vi "运维调试_质控单元.vi"() -> ()   [LabVIEW 2016, in "质控单元.lvlib"]
uses:
  <vilib>/Utility/miscctls.llb/LVPointTypeDef.ctl
  <vilib>/Analysis/6fits.llb/Curve Fitting Criteria.ctl
  <vilib>/Plasmionique/MB Master/MB_Master_Serial/MB_Master_Serial.lvclass
  C:/Program Files (x86)/National Instruments/LabVIEW 2016/vi.lib/Plasmionique/MB Master/MB_Master/MB_Master.lvclass
  <vilib>/Utility/config.llb/Write Key (I32).vi
  <vilib>/Utility/config.llb/Write Key (Double).vi
  <vilib>/Utility/config.llb/Write Key (Boolean).vi
  <vilib>/Utility/config.llb/Write Key (U32).vi
  <vilib>/Utility/config.llb/Read Key (I32).vi
  <vilib>/Utility/config.llb/Read Key (Double).vi
  <vilib>/Utility/config.llb/Read Key (Boolean).vi
  <vilib>/Utility/config.llb/Read Key (U32).vi
  <vilib>/Plasmionique/MB Master/MB Master.lvlib
  <vilib>/ptbypt/NI_PtbyPt.lvlib
  <vilib>/Utility/config.llb/NI_LVConfig.lvlib
  <vilib>/Analysis/NI_AALPro.lvlib
panel:
  out "CODMn质控中断报警":bool
  out "总磷质控中断报警":bool
  out "总氮质控中断报警":bool
  out "氨氮质控中断报警":bool
  in  "报警清除":bool
  in  "CODMn量程选择":enum32{"H", "L", "AUTO"}(ring)
  in  "CODMn加标回收启动":bool
  in  "总磷总氮加标回收启动":bool
  in  "氨氮加标回收启动":bool
  in  "总磷量程选择":enum32{"H", "L", "AUTO"}(ring)=enum."AUTO"
  in  "总氮量程选择":enum32{"H", "L", "AUTO"}(ring)=enum."AUTO"
  in  "氨氮量程选择":enum32{"H", "L", "AUTO"}(ring)=enum."AUTO"
  out "COD超时报警":bool
  out "总磷总氮超时报警":bool
  out "氨氮进样超时报警":bool
  out "簇":T1
  out "通讯指示灯3":bool
  out "通讯指示灯2":bool
  out "通讯指示灯1":bool
  in  "模块选择 3":bool
  in  "模块选择 2":bool
  in  "模块选择":bool
  in  "枚举":enum16{"柱塞泵1", "柱塞泵2", "柱塞泵3"}(ring)
  in  "启用":bool
  in  "B 3":dbl caption="B3"
  in  "K 3":dbl caption="K3"
  in  "B 2":dbl caption="B2"
  in  "K 2":dbl caption="K2"
  in  "B":dbl caption="B1"
  in  "K":dbl caption="K1"
  out "r^2":dbl format="%_6g"
  out "拟合方程":string
  in  "实际体积 5":dbl
  in  "标准体积 5":dbl
  in  "实际体积 4":dbl
  in  "标准体积 4":dbl
  in  "实际体积 3":dbl
  in  "实际体积 2":dbl
  in  "实际体积 1":dbl
  in  "标准体积 3":dbl
  in  "标准体积 2":dbl
  in  "标准体积 1":dbl
  in  "读取":bool
  in  "柱塞泵3":bool
  in  "柱塞泵2":bool
  in  "柱塞泵1":bool
  in  "注出体积选择":u16(ring) items=["0.1mL", "0.3mL", "0.5mL", "0.8mL", "1.0mL"]
  out "Serial Config":T2={"baud rate (bps)"=115200, "stop bits"=10, "parity"=0, "flow control"=0, "timeout"=100, "retries"=1} {"stop bits" items=["1.0"=10, "1.5"=15, "2.0"=20]; "parity" items=["None", "Odd", "Even", "Mark", "Space"]; "flow control" items=["None", "XON/XOFF", "RTS/CTS", "XON/XOFF & RTS/CTS", "DTR/DSR", "XON/XOFF & DTR/DSR"]}
  out "VISA Resource":refnum<visa-resource-name>="COM8"
  in  "背隙补偿步数 3":i32 min=0 max=2000
  in  "背隙补偿步数 2":i32 min=0 max=2000
  in  "写入":bool
  in  "背隙补偿步数":i32 min=0 max=2000
  out "总氮加标回收测完标志":bool
  out "启动模块":T3
  out "COD传感器故障报警":bool
  in  "总氮停止":bool
  in  "总氮排液":bool
  in  "总氮调试":bool
  out "总氮加标回收率":dbl caption="加标回收率" format="%.2f"
  out "总氮加标体积":dbl caption="加标体积" format="%.3f"
  out "总氮母液浓度":dbl caption="加标母液浓度" format="%.3f"
  out "总氮加标水杯定容体积":dbl caption="加标水杯定容体积" format="%.2f"
  out "总氮加标后水样浓度":dbl caption="加标后水样浓度" format="%.3f"
  out "总氮加标前水样浓度":dbl caption="加标前水样浓度" format="%.3f"
  out "总氮检出限":dbl caption="检出限" format="%.3f"
  out "总氮量程":dbl caption="量程" format="%.2f"
  out "总氮状态":u16(ring) caption="状态" items=["待机", "润洗", "进样", "等待取液", "排液"]
  in  "返回":bool
  in  "查看":bool
  out "直接启动":bool
  out "常规启动":bool
  out "总磷总氮传感器故障报警":bool
  out "氨氮传感器故障报警":bool
  out "columns":string[](array[string])
  out "data":T4
  out "氨氮加标回收测完标志":bool
  out "COD加标回收测完标志":bool
  out "总磷加标回收测完标志":bool
  out "COD平行样测完标志":bool
  out "氨氮总磷平行样测完标志":bool
  out "输出簇 2":T5
  out "常规启动 2":bool
  out "直接启动 2":bool
  out "启动模块 2":cluster{"氨氮1":bool, "总磷1":bool, " COD1":bool}
  in  "停止测量":bool
  out "输出簇":T6
  in  "加标回收":bool
  in  "平行样测试":bool
  in  "CODMn停止":bool
  in  "CODMn排液":bool
  in  "CODMn调试":bool
  in  "总磷停止":bool
  in  "总磷排液":bool
  in  "总磷调试":bool
  out "COD加标回收率":dbl caption="加标回收率" format="%.2f"
  out "COD加标体积":dbl caption="加标体积" format="%.3f"
  out "COD母液浓度":dbl caption="加标母液浓度" format="%.2f"
  out "COD加标水杯定容体积":dbl caption="加标水杯定容体积" format="%.2f"
  out "COD加标后水样浓度":dbl caption="加标后水样浓度" format="%.2f"
  out "COD加标前水样浓度":dbl caption="加标前水样浓度" format="%.2f"
  out "COD检出限":dbl caption="检出限" format="%.2f"
  out "COD量程":dbl caption="量程" format="%.2f"
  out "COD状态":u16(ring) caption="状态" items=["待机", "润洗", "进样", "等待取液", "排液"]
  out "总磷加标回收率":dbl caption="加标回收率" format="%.2f"
  out "总磷加标体积":dbl caption="加标体积" format="%.3f"
  out "总磷母液浓度":dbl caption="加标母液浓度" format="%.3f"
  out "总磷加标水杯定容体积":dbl caption="加标水杯定容体积" format="%.2f"
  out "总磷加标后水样浓度":dbl caption="加标后水样浓度" format="%.3f"
  out "总磷加标前水样浓度":dbl caption="加标前水样浓度" format="%.3f"
  out "总磷检出限":dbl caption="检出限" format="%.3f"
  out "总磷量程":dbl caption="量程" format="%.2f"
  out "总磷状态":u16(ring) caption="状态" items=["待机", "润洗", "进样", "等待取液", "排液"]
  out "氨氮加标回收率":dbl caption="加标回收率" format="%.2f"
  out "氨氮加标体积":dbl caption="加标体积" format="%.3f"
  out "氨氮母液浓度":dbl caption="加标母液浓度" format="%.3f"
  out "氨氮加标水杯定容体积":dbl caption="加标水杯定容体积" format="%.2f"
  out "氨氮加标后水样浓度":dbl caption="加标后水样浓度" format="%.3f"
  out "氨氮加标前水样浓度":dbl caption="加标前水样浓度" format="%.3f"
  out "氨氮检出限":dbl caption="检出限" format="%.3f"
  out "氨氮量程":dbl caption="量程" format="%.2f"
  out "氨氮状态":u16(ring) caption="状态" items=["待机", "润洗", "进样", "等待取液", "排液"]
  in  "氨氮停止":bool
  in  "氨氮排液":bool
  in  "氨氮调试":bool
  # "参数配置区"
  # "2000步等于1mL\n100步等于0.05mL\n20步等于0.01mL\n2步等于0.001mL\n（初始默认100步）"
  # "辅助计算区"
  # "状态显示区"
  # "总氮质控参数"
  # "%"
  # "mL"
  # "mg/L"
  # "mL"
  # "mg/L"
  # "mg/L"
  # "mg/L"
  # "mg/L"
  # "CODMn质控参数"
  # "%"
  # "mL"
  # "mg/L"
  # "mL"
  # "mg/L"
  # "mg/L"
  # "mg/L"
  # "mg/L"
  # "总磷质控参数"
  # "%"
  # "mL"
  # "mg/L"
  # "mL"
  # "mg/L"
  # "mg/L"
  # "mg/L"
  # "mg/L"
  # "氨氮质控参数"
  # "%"
  # "mL"
  # "mg/L"
  # "mL"
  # "mg/L"
  # "mg/L"
  # "mg/L"
  # "mg/L"
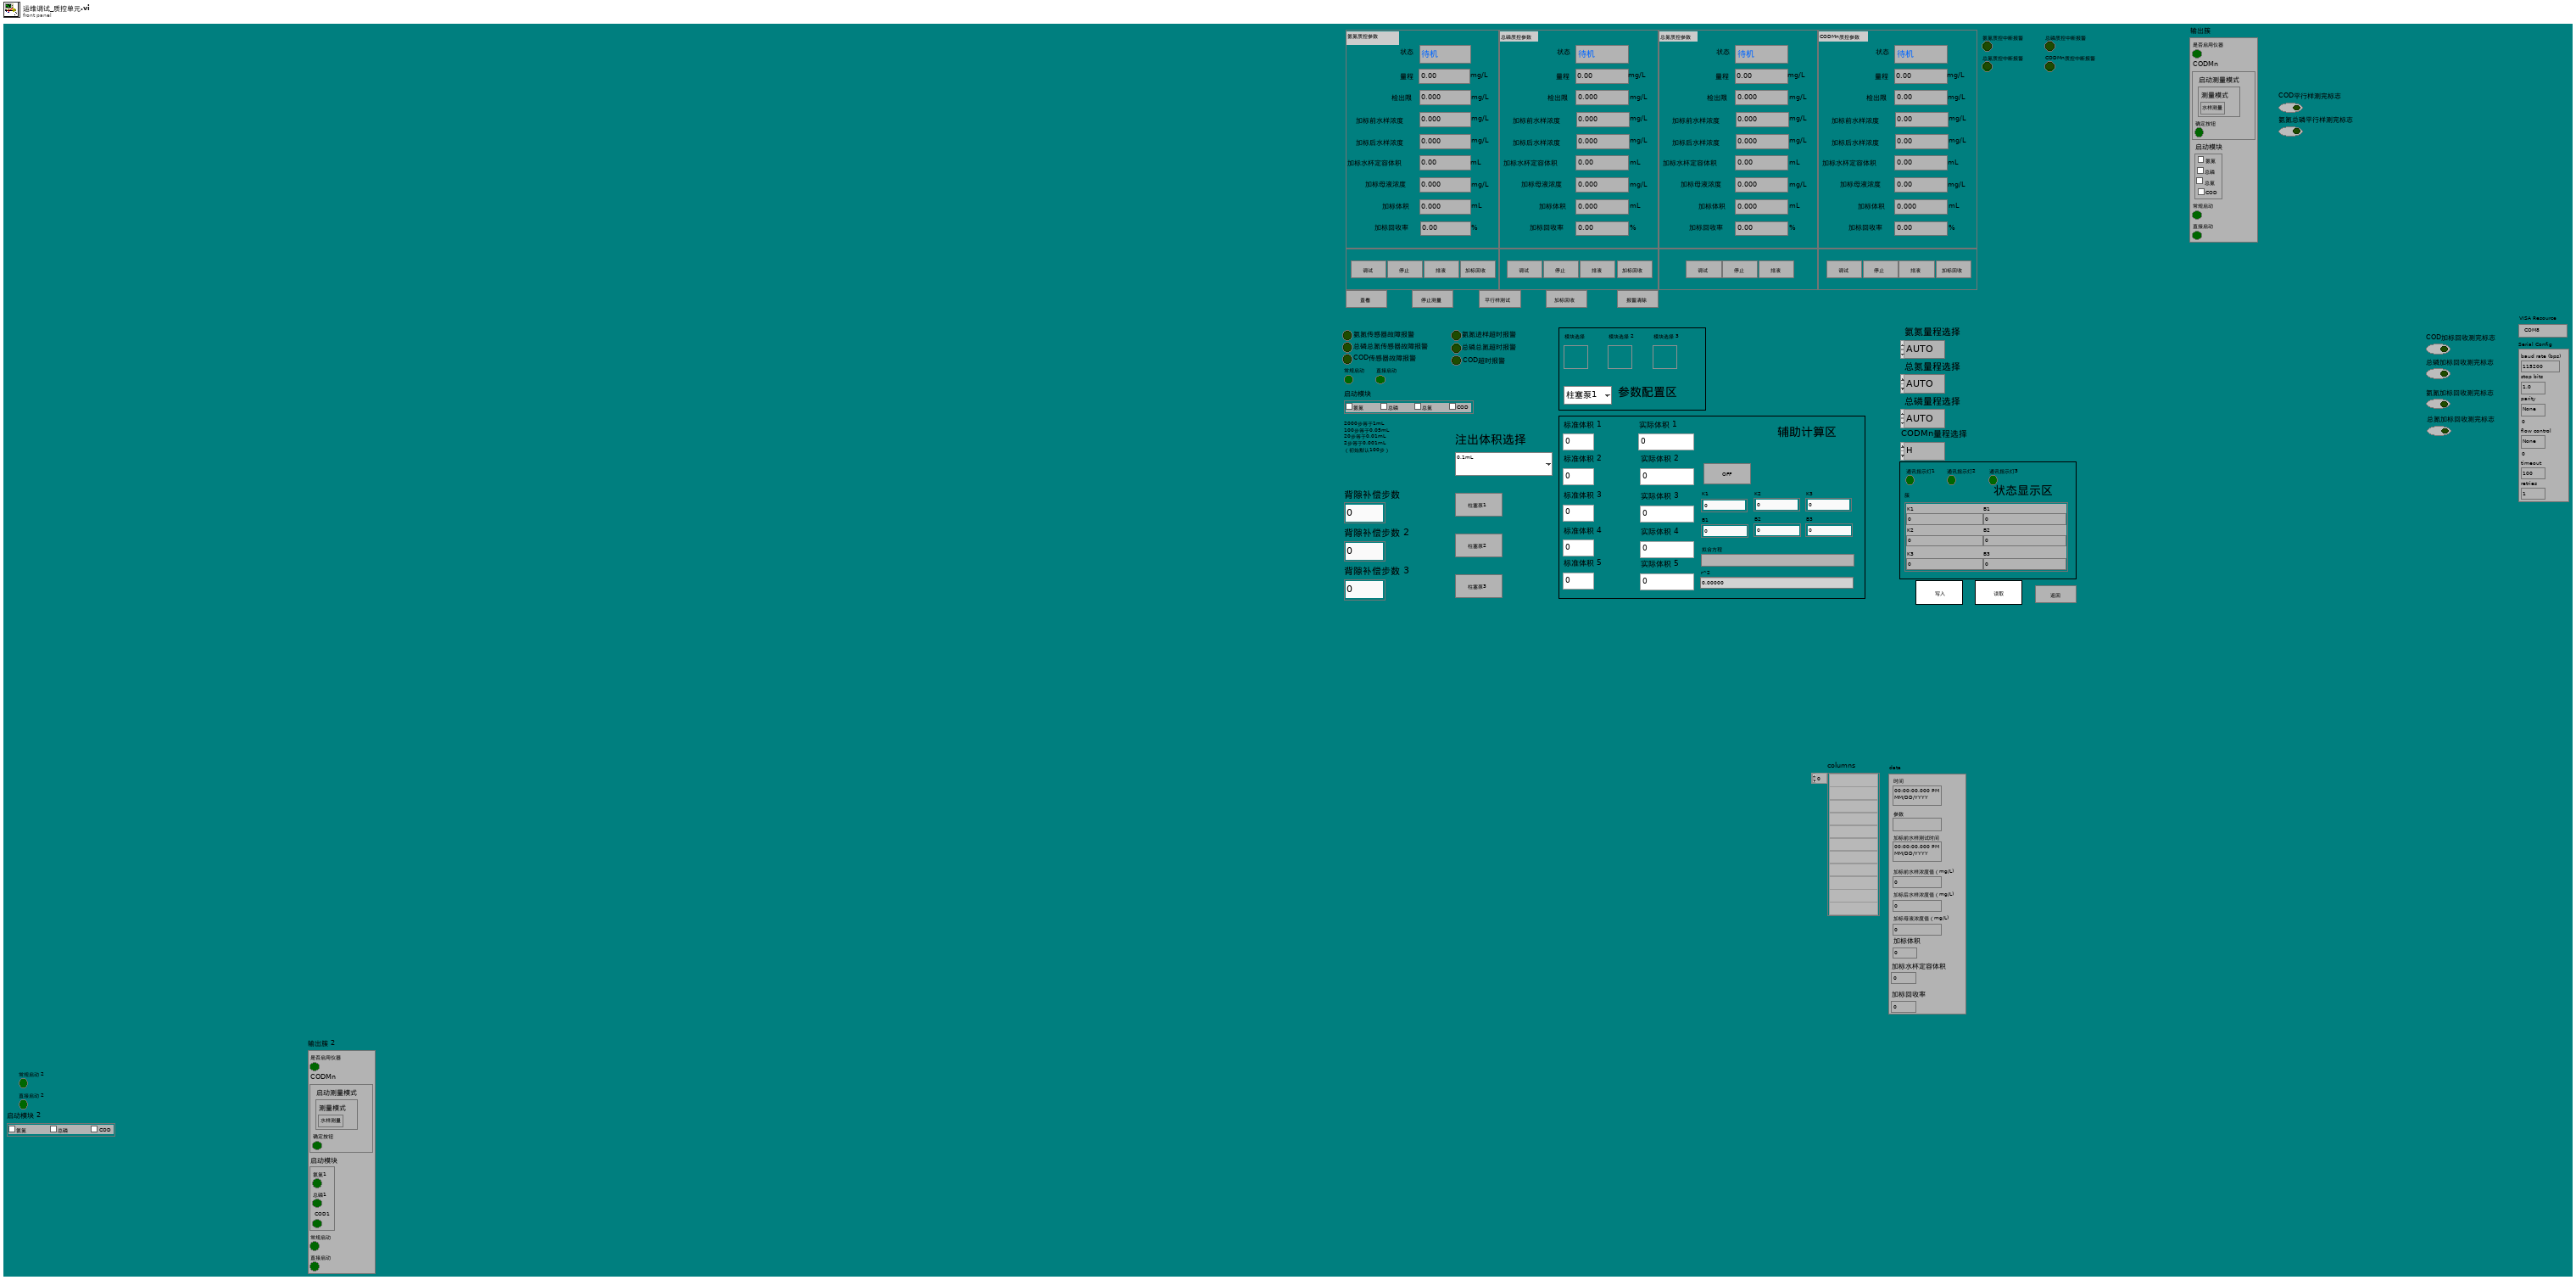
[diagram p1: front panel]
types:
  T1 = cluster{"K1":sgl, "B1":sgl, "K2":sgl, "B2":sgl, "K3":sgl, "B3":sgl}
  T2 = cluster{"baud rate (bps)":u32, "stop bits":u16, "parity":u16, "flow control":u16, "timeout":u32, "retries":i32}
  T3 = cluster{"氨氮":bool, "总磷":bool, "总氮":bool, "COD":bool}
  T4 = cluster{"时间":timestamp, "参数":string, "加标前水样测试时间":timestamp, "加标前水样浓度值（mg/L)":sgl, "加标后水样浓度值（mg/L)":sgl, "加标母液浓度值（mg/L)":sgl, "加标体积":dbl, "加标水杯定容体积":dbl, "加标回收率":dbl}
  T5 = cluster{"是否启用仪器":bool, "CODMn":cluster{"启动测量模式":cluster{"测量模式":enum16{"水样测量", "标样核查", "加标回收", "平行样", "校零", "校标"}}, "确定按钮":bool}, "启动模块":cluster{"氨氮1":bool, "总磷1":bool, " COD1":bool}, "常规启动":bool, "直接启动":bool}
  T6 = cluster{"是否启用仪器":bool, "CODMn":cluster{"启动测量模式":cluster{"测量模式":enum16{"水样测量", "标样核查", "加标回收", "平行样", "校零", "校标"}}, "确定按钮":bool}, "启动模块 3":cluster{"氨氮":bool, "总磷":bool, "总氮":bool, "COD":bool}, "常规启动":bool, "直接启动":bool}
  T7 = typedef "LVPointTypeDef.ctl" = cluster{"Horizontal":i16, "Vertical":i16}
  T8 = cluster{"量程":dbl, "检出限":dbl, "加标前水样浓度":dbl, "加标后水样浓度":dbl, "加标水杯定容体积":dbl, "加标母液浓度":dbl, "加标体积":dbl, "加标回收率":dbl}
  T9 = cluster{"因子编码":u32, "单位":u16, "标样参考值":sgl, "水样数据时间":timestamp, "水样实测值":sgl, "水样数据标识":string, "标样数据时间":timestamp, "标样实测值":sgl, "标样数据标识":string, "空白数据时间":timestamp, "空白实测值":sgl, "空白数据标识":string, "零点核查数据时间":timestamp, "零点核查实测值":sgl, "零点核查数据标识":string, "跨度核查数据时间":timestamp, "跨度核查实测值":sgl, "跨度核查数据标识":string, "加标回收数据时间":timestamp, "加标回收实测值":sgl, "加标回收数据标识":string, "平行样数据时间":timestamp, "平行样实测值":sgl, "平行样数据标识":string}
  T10 = cluster{"因子编码":u32, "单位":u16, "标样参考值":sgl, "水样数据时间":timestamp, "水样实测值":sgl, "水样数据标识":string, "标样数据时间":timestamp, "标样实测值":sgl, "标样数据标识":string, "空白数据时间":timestamp, "空白实测值":sgl, "空白数据标识":string, "零点核查数据时间":timestamp, "零点核查实测值":sgl, "零点核查数据标识":string, "跨度核查数据时间":timestamp, "跨度核查实测值":sgl, "跨度核查数据标识":string, "加标回收数据时间":timestamp, "加标回收实测值":sgl, "加标回收数据标识":string, "平行样数据时间":timestamp, "平行样实测值":sgl, "平行样数据标识":string, "F0":sgl, "F1":sgl, "F2":sgl, "F3":sgl, "F4":sgl, "F5":sgl, "F6":sgl, "F7":sgl, "温度":sgl, "湿度":sgl, "X值":sgl}
  T11 = enum8{"Enabled", "Disabled", "Disabled and Grayed Out"}
  T12 = typedef "NI_AALPro.lvlib/Curve Fitting Criteria.ctl" = u16
  T13 = typedef "NI_LVConfig.lvlib/Config Data RefNum.ctl" = refnum<k1>
  T14 = cluster{"命令":string, cluster{"starting address":u16, "holding register value":u16}}
  T15 = enum32{"Bad", "Idle", "Run top level", "Running"}
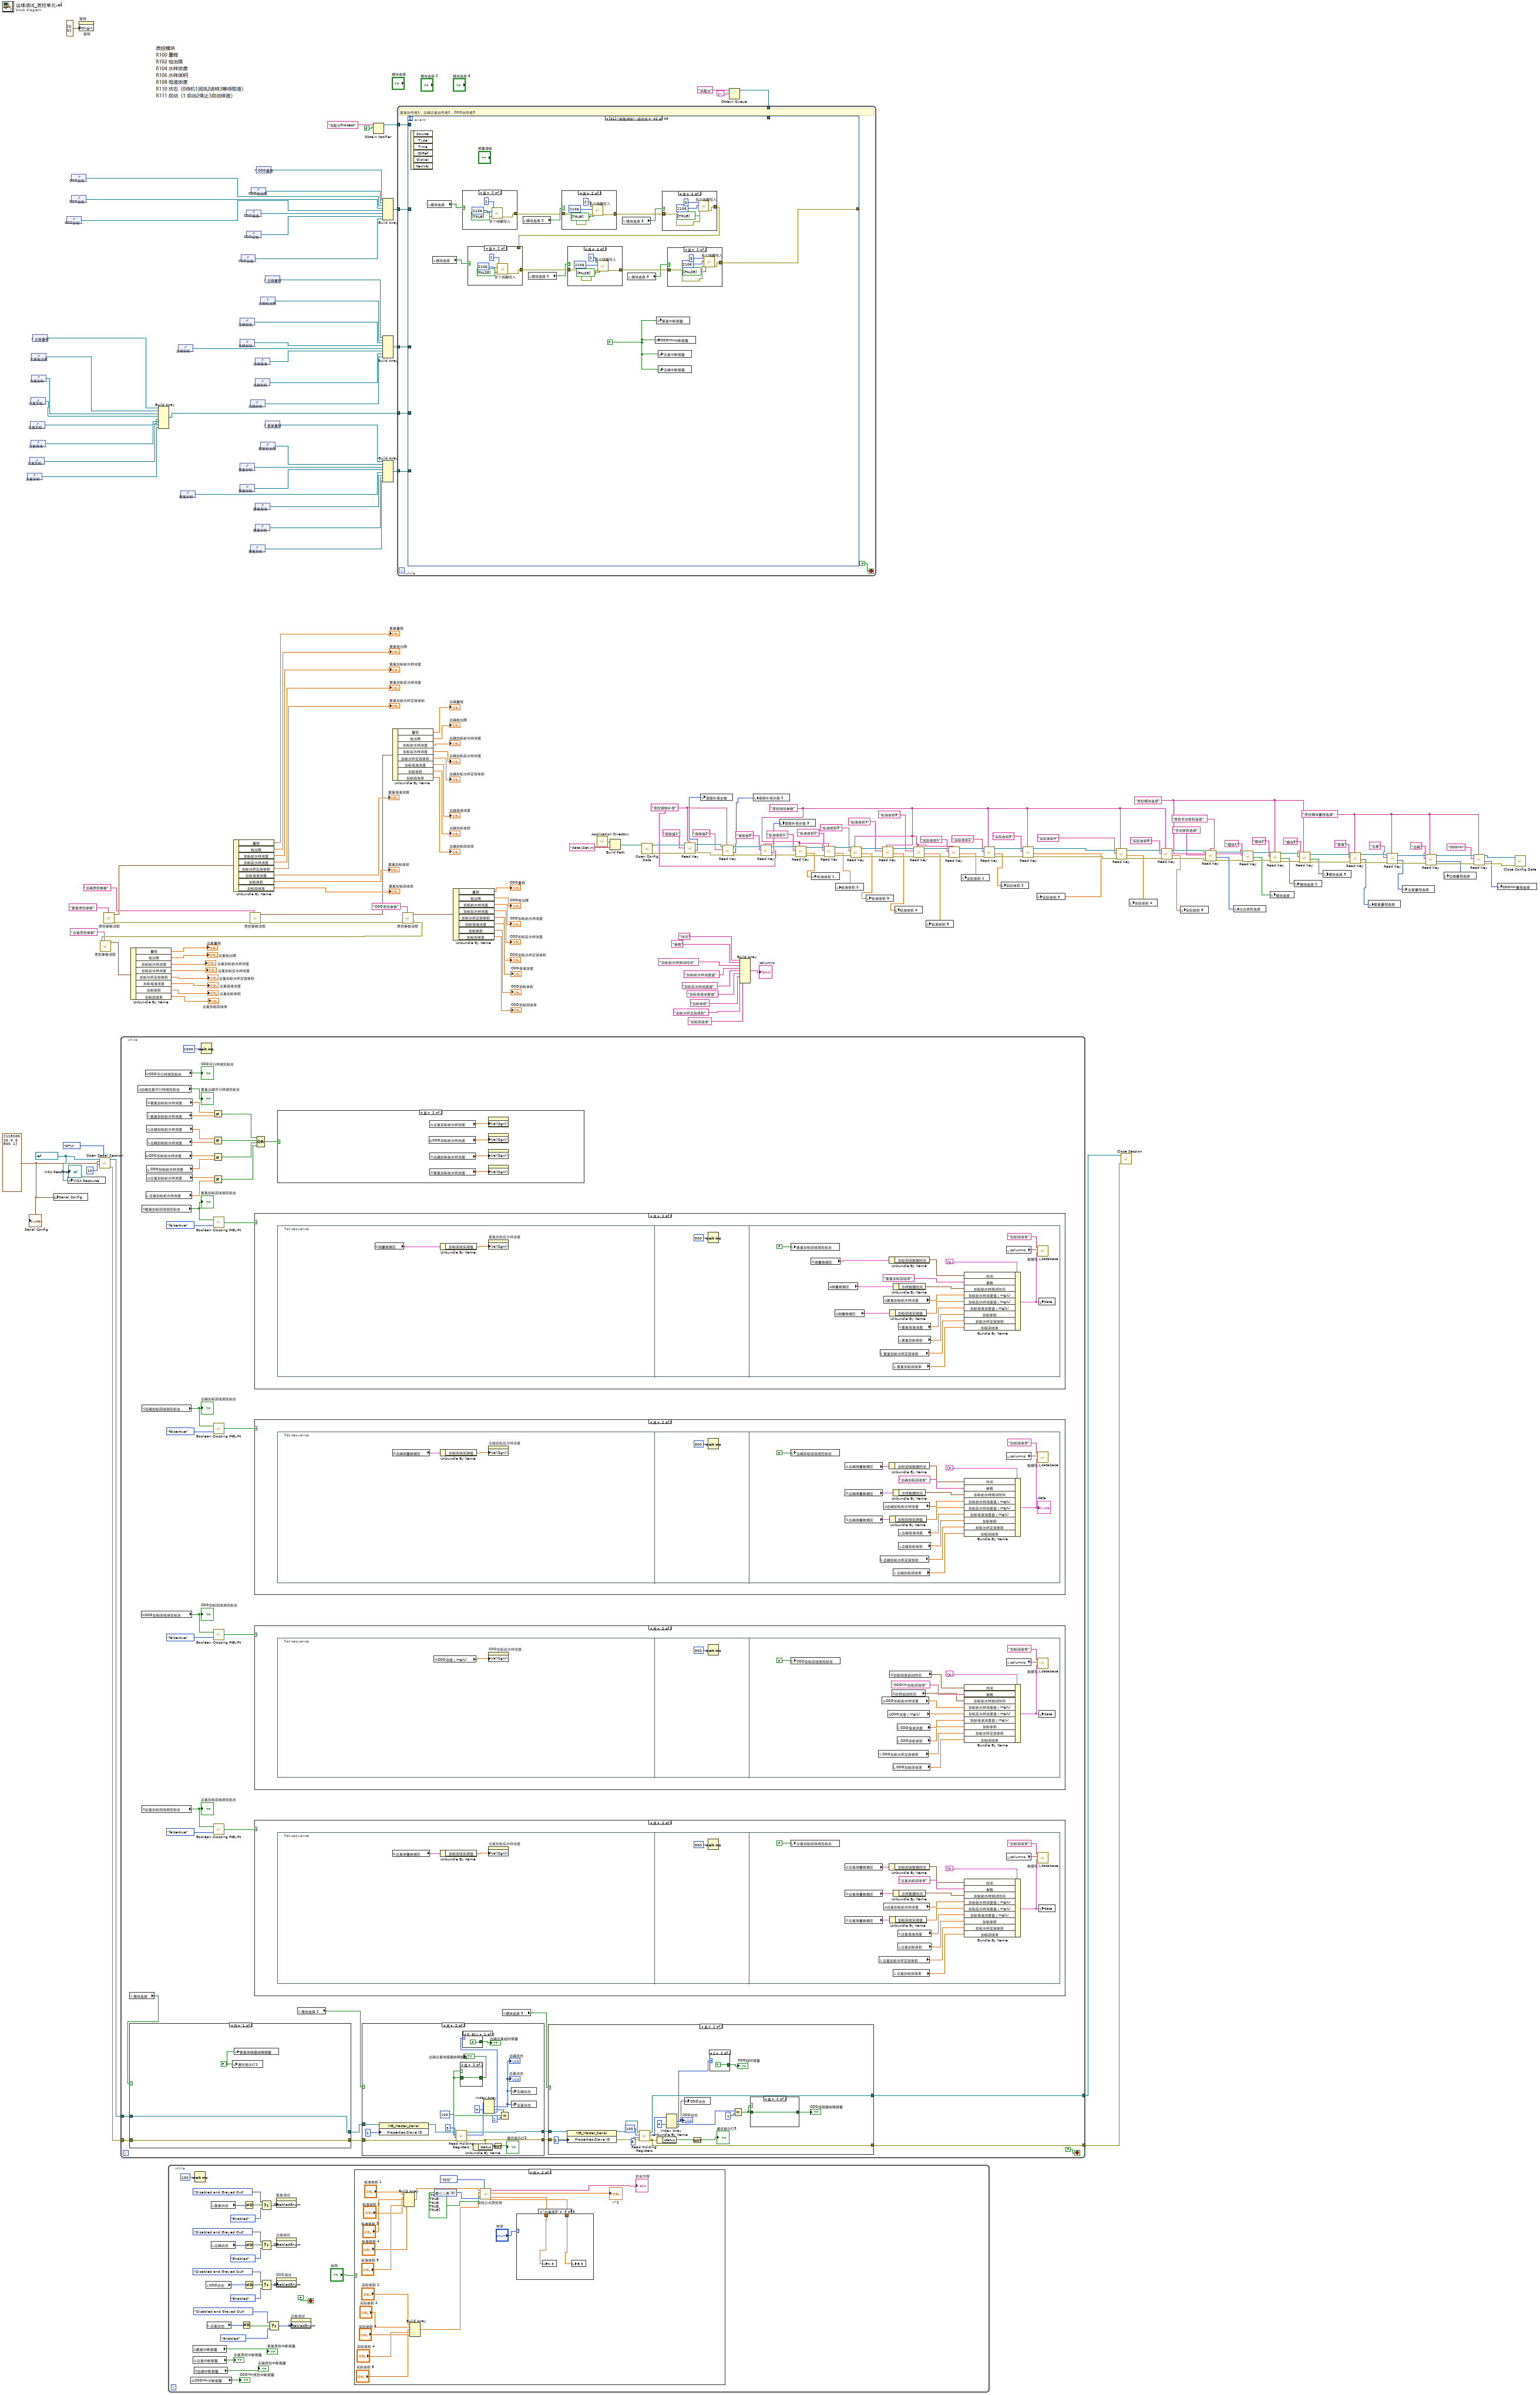
[diagram p0: block diagram]
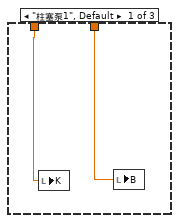
[diagram p3: hidden frame]
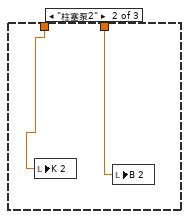
[diagram p4: hidden frame]
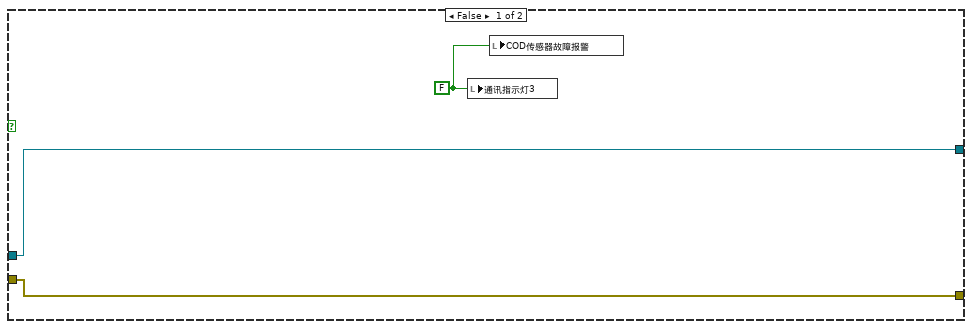
[diagram p5: hidden frame]
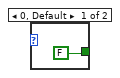
[diagram p6: hidden frame]
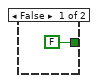
[diagram p7: hidden frame]
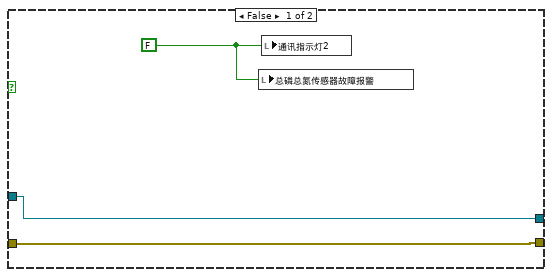
[diagram p8: hidden frame]
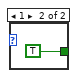
[diagram p9: hidden frame]
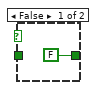
[diagram p10: hidden frame]
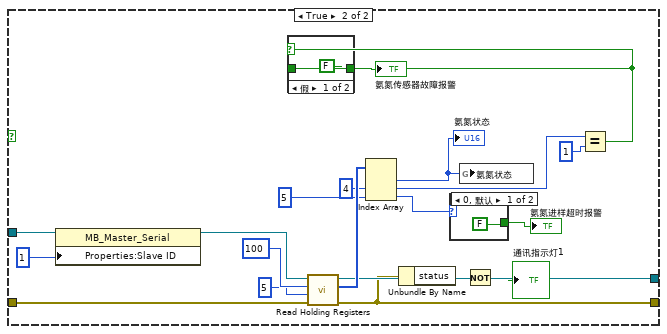
[diagram p11: hidden frame]
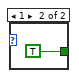
[diagram p12: hidden frame]
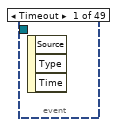
[diagram p19: hidden frame]
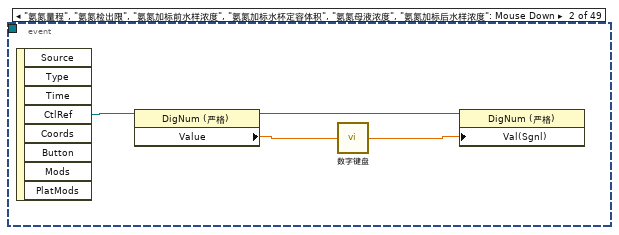
[diagram p20: hidden frame]
diagram:
  w17 = "质控模块量程选择" ("section")
  w32 = "质控模块选择" ("section")
  w70 = "质控线性参数" ("section")
  w88 = "质控背隙补偿" ("section")
  w95 = T2 {"baud rate (bps)"=115200, "stop bits"=10, "parity"=0, "flow control"=0, "timeout"=500, "retries"=1} ("Serial Config")
  w96 = refnum<visa-resource-name> "COM8" ("VISA Resource")
  n1 = control-ref of="总氮加标回收率"() -> (w113:refnum<vi>)
  n2 = control-ref of="总氮加标体积"() -> (w114:refnum<vi>)
  n3 = control-ref of="总氮加标水杯定容体积"() -> (w116:refnum<vi>)
  n4 = control-ref of="总氮加标后水样浓度"() -> (w117:refnum<vi>)
  n5 = control-ref of="总氮母液浓度"() -> (w115:refnum<vi>)
  n6 = control-ref of="总氮检出限"() -> (w119:refnum<vi>)
  n7 = control-ref of="总氮加标前水样浓度"() -> (w118:refnum<vi>)
  n8 = control-ref of="总氮量程"() -> (w120:refnum<vi>)
  n9 = global write "串口参数全局.vi" "Serial Config"(w95) -> ()
  n10 = control-ref of="COD加标水杯定容体积"() -> (w144:refnum<vi>)
  n11 = global write "串口参数全局.vi" "VISA Resource"(w96) -> ()
  n12 = control-ref of="COD加标前水样浓度"() -> (w146:refnum<vi>)
  n13 = control-ref of="COD加标后水样浓度"() -> (w145:refnum<vi>)
  n14 = property on="窗格" class="Pane"("Origin"=T7 {"Horizontal"=0, "Vertical"=0} ("原点")) -> ()  [unwired: 2 in, 2 out]
  n15 = property on="窗格" class="Pane"("Origin"=T7 {"Horizontal"=0, "Vertical"=0} ("原点")) -> ()  [unwired: 2 in, 2 out]
  n16 = call <vilib>:"Open Serial Session.vi"("Mode (RTU)"=enum16{"RTU", "ASCII"}."RTU", "Slave ID"=u8 10, "Serial Config"=w95, "VISA Resource"=w96) -> ("Error out"=w138:errorcluster, "MB_Serial session"=w139:refnum<class "MB_Master_Serial.lvclass">)  [unwired: 6 in]
  n17 = call "质控参数读取.vi"("section"="氨氮质控参数") -> ("error out"=w169:errorcluster, "参数"=w188:T8)  [unwired: 9 in]
  n18 = while {
    tunnel: w139 -> [w237]
    tunnel: w138 -> [w236]
    tunnel: [w203] -> w137
    tunnel: [w212] -> w97
    stop <- FALSE stop-if-true
    n19 = local read "模块选择"() -> (w202:bool)
    n20 = case shown="假" w202 {
      tunnel: w237 -> [w294 w314]
      tunnel: w236 -> [w293 w313]
      tunnel: [w294 w301] -> w207
      tunnel: [w293 w300] -> w205
      frame False {
        w292 = FALSE ("通讯指示灯1")
        n21 = local write "通讯指示灯1"(w292) -> ()
        n22 = local write "氨氮传感器故障报警"(w292) -> ()
      }
      frame True {
        n23 = property class="MB_Master_Serial"(reference=w314, "Properties:Slave ID"=u8 1 ("Slave ID")) -> (reference out=w309:refnum<class "MB_Master_Serial.lvclass">)  [unwired: 1 in, 1 out]
        n24 = call <vilib>:"Read Holding Registers.vi"("error in (no error)"=w313, "quantity"=u16 5, "starting address"=u16 100, "MB session in"=w309) -> ("error out"=w300:errorcluster, "Registers"=w310:u16[], "MB session out"=w301:refnum<class "MB_Master_Serial.lvclass">)  [unwired: 5 in]
        n25 = Index Array(array=w310, index #2=4 ("索引"), index #3=5 ("索引")) -> (element #1=w302:u16, element #2=w306:u16, element #3=w296:u16)  [unwired: 1 in]
        "氨氮状态" <- w302
        n26 = Unbundle By Name(w300) -> ("status"=w299:bool)
        n27 = case shown="0, 默认" w296 {
          tunnel: [FALSE TRUE] -> w295
          frame 0, Default {
          }
          frame 1 {
          }
        }
        "氨氮进样超时报警" <- w295
        n28 = global write "氨氮加标回收状态全局变量.vi" "氨氮状态"(w302) -> ()
        n29 = Not(x=w299) -> (.not. x?=→"通讯指示灯1":bool)
        n30 = Equal?(x=w306, y=u16 1) -> (x = y?=w303:bool)
        n31 = case shown="假" w303 {
          tunnel: w303 -> [_ w318]
          tunnel: [FALSE w318] -> w304
          frame False {
          }
          frame True {
          }
        }
        "氨氮传感器故障报警" <- w304
      }
    }
    n32 = global read "质控测完标志全局 1.vi" "总磷总氮平行样测完标志"() -> (→"氨氮总磷平行样测完标志":bool)
    n33 = global read "质控测完标志全局 1.vi" "COD加标回收测完标志"() -> (w218:bool)
    "COD加标回收测完标志" <- w218
    n34 = global read "质控测完标志全局 1.vi" "氨氮加标回收测完标志"() -> (w223:bool)
    "氨氮加标回收测完标志" <- w223
    n35 = global read "质控测完标志全局 1.vi" "总磷加标回收测完标志"() -> (w211:bool)
    "总磷加标回收测完标志" <- w211
    n36 = global read "质控测完标志全局 1.vi" "总氮加标回收测完标志"() -> (w209:bool)
    "总氮加标回收测完标志" <- w209
    n37 = global read "质控测完标志全局 1.vi" "COD平行样测完标志"() -> (→"COD平行样测完标志":bool)
    n38 = global read "水样浓度全局.vi" "COD加标前水样浓度"() -> (w231:dbl)
    n39 = local read "总氮加标前水样浓度"() -> (w215:dbl)
    n40 = global read "水样浓度全局.vi" "氨氮加标前水样浓度"() -> (w235:dbl)
    n41 = global read "水样浓度全局.vi" "总磷加标前水样浓度"() -> (w233:dbl)
    n42 = local read "COD加标前水样浓度"() -> (w230:dbl)
    n43 = global read "水样浓度全局.vi" "总氮加标前水样浓度"() -> (w214:dbl)
    n44 = local read "氨氮加标前水样浓度"() -> (w234:dbl)
    n45 = local read "总磷加标前水样浓度"() -> (w232:dbl)
    n46 = Wait (ms)(milliseconds to wait=u32 1000 ("等待时间（毫秒）")) -> ()  [unwired: 1 out]
    n47 = Not Equal?(x=w235, y=w234) -> (x != y?=w229:bool)
    n48 = Not Equal?(x=w233, y=w232) -> (x != y?=w227:bool)
    n49 = Not Equal?(x=w231, y=w230) -> (x != y?=w226:bool)
    n50 = Not Equal?(x=w214, y=w215) -> (x != y?=w213:bool)
    n51 = call <vilib>:"Boolean Crossing PtByPt.vi"("direction"=enum16{"either", "false-true", "true-false"}."false-true", "input"=w223) -> ("crossing"=w222:bool)  [unwired: 1 in]
    n52 = call <vilib>:"Boolean Crossing PtByPt.vi"("direction"=enum16{"either", "false-true", "true-false"}."false-true", "input"=w211) -> ("crossing"=w219:bool)  [unwired: 1 in]
    n53 = call <vilib>:"Boolean Crossing PtByPt.vi"("direction"=enum16{"either", "false-true", "true-false"}."false-true", "input"=w218) -> ("crossing"=w216:bool)  [unwired: 1 in]
    n54 = call <vilib>:"Boolean Crossing PtByPt.vi"("direction"=enum16{"either", "false-true", "true-false"}."false-true", "input"=w209) -> ("crossing"=w208:bool)  [unwired: 1 in]
    n55 = case shown="真" w222 {
      frame False {
      }
      frame True {
        n56 = flat-sequence {
          frame #0 {
            n57 = global read "VAR总磷氨氮全局变量.vi" "测量数据区"() -> (w375:T9)
            n58 = Unbundle By Name(w375) -> ("加标回收实测值"=w376:sgl)
            n59 = property on="氨氮加标后水样浓度" class="DigNum (严格)"("Val(Sgnl)"=w376) -> ()  [unwired: 2 in, 2 out]
          }
          frame #1 {
            n60 = Wait (ms)(milliseconds to wait=u32 500 ("等待时间（毫秒）")) -> ()  [unwired: 1 out]
          }
          frame #2 {
            n61 = local write "氨氮加标回收测完标志"(FALSE ("氨氮加标回收测完标志")) -> ()
            n62 = global read "VAR总磷氨氮全局变量.vi" "测量数据区"() -> (w380:T9)
            n63 = global read "VAR总磷氨氮全局变量.vi" "测量数据区"() -> (w379:T9)
            n64 = global read "VAR总磷氨氮全局变量.vi" "测量数据区"() -> (w378:T9)
            n65 = local read "氨氮加标水杯定容体积"() -> (w388:dbl)
            n66 = global read "水样浓度全局.vi" "氨氮加标前水样浓度"() -> (w392:dbl)
            n67 = Unbundle By Name(w380) -> ("加标回收数据时间"=w385:timestamp)
            n68 = Unbundle By Name(w378) -> ("加标回收实测值"=w391:sgl)
            n69 = Unbundle By Name(w379) -> ("水样数据时间"=w383:timestamp)
            n70 = local read "氨氮加标回收率"() -> (w387:dbl)
            n71 = local read "氨氮母液浓度"() -> (w390:dbl)
            n72 = local read "氨氮加标体积"() -> (w389:dbl)
            n73 = Bundle By Name(cluster=T4 {"时间"=timestamp(0 s since 1904-01-01), "参数"="", "加标前水样测试时间"=timestamp(0 s since 1904-01-01), "加标前水样浓度值（mg/L)"=0.0, "加标后水样浓度值（mg/L)"=0.0, "加标母液浓度值（mg/L)"=0.0, "加标体积"=0.0, "加标水杯定容体积"=0.0, "加标回收率"=0.0} ("data"), "时间"=w385, "参数"="氨氮加标回收率" ("table"), "加标前水样测试时间"=w383, "加标前水样浓度值（mg/L)"=w392, "加标后水样浓度值（mg/L)"=w391, "加标母液浓度值（mg/L)"=w390, "加标体积"=w389, "加标水杯定容体积"=w388, "加标回收率"=w387) -> (w382:T4)
            n74 = local read "columns"() -> (w393:string[])
            n75 = call "数据写入database.vi"("data"=w382, "columns"=w393, "table"="加标回收率") -> ()  [unwired: 8 in, 1 out]
            n76 = local write "data"(w382) -> ()
          }
        }
      }
    }
    n77 = case shown="真" w219 {
      frame False {
      }
      frame True {
        n78 = flat-sequence {
          frame #0 {
            n79 = global read "VAR总磷氨氮全局变量.vi" "总磷测量数据区"() -> (w356:T10)
            n80 = Unbundle By Name(w356) -> ("加标回收实测值"=w355:sgl)
            n81 = property on="总磷加标后水样浓度" class="DigNum (严格)"("Val(Sgnl)"=w355) -> ()  [unwired: 2 in, 2 out]
          }
          frame #1 {
            n82 = Wait (ms)(milliseconds to wait=u32 500 ("等待时间（毫秒）")) -> ()  [unwired: 1 out]
          }
          frame #2 {
            n83 = local write "总磷加标回收测完标志"(FALSE ("氨氮总磷加标回收测完标志")) -> ()
            n84 = global read "VAR总磷氨氮全局变量.vi" "总磷测量数据区"() -> (w364:T10)
            n85 = global read "VAR总磷氨氮全局变量.vi" "总磷测量数据区"() -> (w360:T10)
            n86 = global read "VAR总磷氨氮全局变量.vi" "总磷测量数据区"() -> (w371:T10)
            n87 = local read "总磷加标水杯定容体积"() -> (w367:dbl)
            n88 = global read "水样浓度全局.vi" "总磷加标前水样浓度"() -> (w372:dbl)
            n89 = Unbundle By Name(w364) -> ("加标回收数据时间"=w361:timestamp)
            n90 = Unbundle By Name(w371) -> ("加标回收实测值"=w370:sgl)
            n91 = Unbundle By Name(w360) -> ("水样数据时间"=w359:timestamp)
            n92 = local read "总磷加标回收率"() -> (w366:dbl)
            n93 = local read "总磷母液浓度"() -> (w369:dbl)
            n94 = local read "总磷加标体积"() -> (w368:dbl)
            n95 = Bundle By Name(cluster=T4 {"时间"=timestamp(0 s since 1904-01-01), "参数"="", "加标前水样测试时间"=timestamp(0 s since 1904-01-01), "加标前水样浓度值（mg/L)"=0.0, "加标后水样浓度值（mg/L)"=0.0, "加标母液浓度值（mg/L)"=0.0, "加标体积"=0.0, "加标水杯定容体积"=0.0, "加标回收率"=0.0} ("data"), "时间"=w361, "参数"="总磷加标回收率" ("table"), "加标前水样测试时间"=w359, "加标前水样浓度值（mg/L)"=w372, "加标后水样浓度值（mg/L)"=w370, "加标母液浓度值（mg/L)"=w369, "加标体积"=w368, "加标水杯定容体积"=w367, "加标回收率"=w366) -> (w365:T4)
            "data" <- w365
            n96 = local read "columns"() -> (w373:string[])
            n97 = call "数据写入database.vi"("data"=w365, "columns"=w373, "table"="加标回收率") -> ()  [unwired: 8 in, 1 out]
          }
        }
      }
    }
    n98 = case shown="真" w216 {
      frame False {
      }
      frame True {
        n99 = flat-sequence {
          frame #0 {
            n100 = global read "COD浓度全局变量.vi" "COD浓度（mg/L)"() -> (w339:dbl)
            n101 = property on="COD加标后水样浓度" class="DigNum (严格)"("Val(Sgnl)"=w339) -> ()  [unwired: 2 in, 2 out]
          }
          frame #1 {
            n102 = Wait (ms)(milliseconds to wait=u32 500 ("等待时间（毫秒）")) -> ()  [unwired: 1 out]
          }
          frame #2 {
            n103 = local write "COD加标回收测完标志"(FALSE ("COD加标回收测完标志")) -> ()
            n104 = local read "COD加标水杯定容体积"() -> (w348:dbl)
            n105 = global read "水样浓度全局.vi" "COD加标前水样浓度"() -> (w352:dbl)
            n106 = global read "COD浓度全局变量.vi" "COD浓度（mg/L)"() -> (w351:dbl)
            n107 = global read "COD测量模式全局.vi" "加标回收启动时间"() -> (w342:timestamp)
            n108 = global read "COD测量模式全局.vi" "水样启动时间"() -> (w341:timestamp)
            n109 = local read "COD加标回收率"() -> (w347:dbl)
            n110 = local read "COD母液浓度"() -> (w350:dbl)
            n111 = local read "COD加标体积"() -> (w349:dbl)
            n112 = Bundle By Name(cluster=T4 {"时间"=timestamp(0 s since 1904-01-01), "参数"="", "加标前水样测试时间"=timestamp(0 s since 1904-01-01), "加标前水样浓度值（mg/L)"=0.0, "加标后水样浓度值（mg/L)"=0.0, "加标母液浓度值（mg/L)"=0.0, "加标体积"=0.0, "加标水杯定容体积"=0.0, "加标回收率"=0.0} ("data"), "时间"=w342, "参数"="CODMn加标回收率" ("table"), "加标前水样测试时间"=w341, "加标前水样浓度值（mg/L)"=w352, "加标后水样浓度值（mg/L)"=w351, "加标母液浓度值（mg/L)"=w350, "加标体积"=w349, "加标水杯定容体积"=w348, "加标回收率"=w347) -> (w346:T4)
            n113 = local read "columns"() -> (w353:string[])
            n114 = call "数据写入database.vi"("data"=w346, "columns"=w353, "table"="加标回收率") -> ()  [unwired: 8 in, 1 out]
            n115 = local write "data"(w346) -> ()
          }
        }
      }
    }
    n116 = case shown="真" w208 {
      frame False {
      }
      frame True {
        n117 = flat-sequence {
          frame #0 {
            n118 = global read "VAR总磷氨氮全局变量.vi" "总氮测量数据区"() -> (w320:T10)
            n119 = Unbundle By Name(w320) -> ("加标回收实测值"=w319:sgl)
            n120 = property on="总氮加标后水样浓度" class="DigNum (严格)"("Val(Sgnl)"=w319) -> ()  [unwired: 2 in, 2 out]
          }
          frame #1 {
            n121 = Wait (ms)(milliseconds to wait=u32 500 ("等待时间（毫秒）")) -> ()  [unwired: 1 out]
          }
          frame #2 {
            n122 = local write "总氮加标回收测完标志"(FALSE ("COD加标回收测完标志")) -> ()
            n123 = global read "VAR总磷氨氮全局变量.vi" "总氮测量数据区"() -> (w329:T10)
            n124 = global read "VAR总磷氨氮全局变量.vi" "总氮测量数据区"() -> (w325:T10)
            n125 = global read "VAR总磷氨氮全局变量.vi" "总氮测量数据区"() -> (w335:T10)
            n126 = local read "总氮加标水杯定容体积"() -> (w331:dbl)
            n127 = global read "水样浓度全局.vi" "总氮加标前水样浓度"() -> (w336:dbl)
            n128 = Unbundle By Name(w329) -> ("加标回收数据时间"=w326:timestamp)
            n129 = Unbundle By Name(w335) -> ("加标回收实测值"=w334:sgl)
            n130 = Unbundle By Name(w325) -> ("水样数据时间"=w324:timestamp)
            n131 = local read "总氮加标回收率"() -> (w330:dbl)
            n132 = local read "总氮母液浓度"() -> (w333:dbl)
            n133 = local read "总氮加标体积"() -> (w332:dbl)
            n134 = Bundle By Name(cluster=T4 {"时间"=timestamp(0 s since 1904-01-01), "参数"="", "加标前水样测试时间"=timestamp(0 s since 1904-01-01), "加标前水样浓度值（mg/L)"=0.0, "加标后水样浓度值（mg/L)"=0.0, "加标母液浓度值（mg/L)"=0.0, "加标体积"=0.0, "加标水杯定容体积"=0.0, "加标回收率"=0.0} ("data"), "时间"=w326, "参数"="总氮加标回收率" ("table"), "加标前水样测试时间"=w324, "加标前水样浓度值（mg/L)"=w336, "加标后水样浓度值（mg/L)"=w334, "加标母液浓度值（mg/L)"=w333, "加标体积"=w332, "加标水杯定容体积"=w331, "加标回收率"=w330) -> (w323:T4)
            n135 = local read "columns"() -> (w337:string[])
            n136 = call "数据写入database.vi"("data"=w323, "columns"=w337, "table"="加标回收率") -> ()  [unwired: 8 in, 1 out]
            n137 = local write "data"(w323) -> ()
          }
        }
      }
    }
    n138 = Compound Arithmetic op=OR ("复合运算")(w229, w227, w226, w213) -> (w228:bool)
    n139 = case shown="真" w228 {
      frame False {
      }
      frame True {
        n140 = global read "水样浓度全局.vi" "COD加标前水样浓度"() -> (w396:dbl)
        n141 = global read "水样浓度全局.vi" "总氮加标前水样浓度"() -> (w395:dbl)
        n142 = global read "水样浓度全局.vi" "总磷加标前水样浓度"() -> (w397:dbl)
        n143 = global read "水样浓度全局.vi" "氨氮加标前水样浓度"() -> (w398:dbl)
        n144 = property on="总氮加标前水样浓度" class="DigNum (严格)"("Val(Sgnl)"=w395) -> ()  [unwired: 2 in, 2 out]
        n145 = property on="COD加标前水样浓度" class="DigNum (严格)"("Val(Sgnl)"=w396) -> ()  [unwired: 2 in, 2 out]
        n146 = property on="总磷加标前水样浓度" class="DigNum (严格)"("Val(Sgnl)"=w397) -> ()  [unwired: 2 in, 2 out]
        n147 = property on="氨氮加标前水样浓度" class="DigNum (严格)"("Val(Sgnl)"=w398) -> ()  [unwired: 2 in, 2 out]
      }
    }
    n148 = local read "模块选择 2"() -> (w201:bool)
    n149 = case shown="真" w201 {
      tunnel: w207 -> [w268 w276]
      tunnel: [w268 w275] -> w206
      tunnel: w205 -> [w267 w274]
      tunnel: [w267 w272] -> w204
      frame False {
        w266 = FALSE ("通讯指示灯2")
        n150 = local write "总磷总氮传感器故障报警"(w266) -> ()
        n151 = local write "通讯指示灯2"(w266) -> ()
      }
      frame True {
        n152 = property class="MB_Master_Serial"(reference=w276, "Properties:Slave ID"=u8 2 ("Slave ID")) -> (reference out=w284:refnum<class "MB_Master_Serial.lvclass">)  [unwired: 1 in, 1 out]
        n153 = call <vilib>:"Read Holding Registers.vi"("error in (no error)"=w274, "quantity"=u16 5, "starting address"=u16 100, "MB session in"=w284) -> ("error out"=w272:errorcluster, "Registers"=w287:u16[], "MB session out"=w275:refnum<class "MB_Master_Serial.lvclass">)  [unwired: 5 in]
        n154 = Unbundle By Name(w272) -> ("status"=w273:bool)
        n155 = Index Array(array=w287, index #2=4 ("索引")) -> (element #1=w277:u16, element #2=w280:u16, element #3=w269:u16)  [unwired: 2 in]
        "总磷状态" <- w277
        "总氮状态" <- w277
        n156 = case shown="0, 默认" w269 {
          tunnel: [FALSE TRUE] -> w270
          frame 0, Default {
          }
          frame 1 {
          }
        }
        "总磷总氮超时报警" <- w270
        n157 = Not(x=w273) -> (.not. x?=→"通讯指示灯2":bool)
        n158 = Equal?(x=w280, y=u16 1) -> (x = y?=w278:bool)
        n159 = case shown="真" w278 {
          tunnel: w278 -> [_ w291]
          tunnel: [FALSE w291] -> w279
          frame False {
          }
          frame True {
          }
        }
        "总磷总氮传感器故障报警" <- w279
        n160 = global write "氨氮加标回收状态全局变量.vi" "总磷状态"(w277) -> ()
        n161 = global write "氨氮加标回收状态全局变量.vi" "总氮状态"(w277) -> ()
      }
    }
    n162 = local read "模块选择 3"() -> (w200:bool)
    n163 = case shown="真" w200 {
      tunnel: [w242 w257] -> w212
      tunnel: w206 -> [w242 w249]
      tunnel: w204 -> [w241 w248]
      tunnel: [w241 w246] -> w203
      frame False {
        w240 = FALSE ("通讯指示灯3")
        n164 = local write "通讯指示灯3"(w240) -> ()
        n165 = local write "COD传感器故障报警"(w240) -> ()
      }
      frame True {
        n166 = property class="MB_Master_Serial"(reference=w249, "Properties:Slave ID"=u8 3 ("Slave ID")) -> (reference out=w260:refnum<class "MB_Master_Serial.lvclass">)  [unwired: 1 in, 1 out]
        n167 = call <vilib>:"Read Holding Registers.vi"("error in (no error)"=w248, "quantity"=u16 5, "starting address"=u16 100, "MB session in"=w260) -> ("error out"=w246:errorcluster, "Registers"=w256:u16[], "MB session out"=w257:refnum<class "MB_Master_Serial.lvclass">)  [unwired: 5 in]
        n168 = Unbundle By Name(w246) -> ("status"=w247:bool)
        n169 = Index Array(array=w256, index #2=4 ("索引")) -> (element #1=w254:u16, element #2=w251:u16, element #3=w243:u16)  [unwired: 2 in]
        "COD状态" <- w254
        n170 = global write "氨氮加标回收状态全局变量.vi" "COD状态"(w254) -> ()
        n171 = Not(x=w247) -> (.not. x?=→"通讯指示灯3":bool)
        n172 = case shown="1" w243 {
          tunnel: [FALSE TRUE] -> w244
          frame 0, Default {
          }
          frame 1 {
          }
        }
        "COD超时报警" <- w244
        n173 = Equal?(x=w251, y=u16 1) -> (x = y?=w253:bool)
        n174 = case shown="真" w253 {
          tunnel: w253 -> [_ w265]
          tunnel: [FALSE w265] -> w250
          frame False {
          }
          frame True {
          }
        }
        "COD传感器故障报警" <- w250
      }
    }
  }
  n175 = Build Array(w120, w119, w118, w117, w116, w115, w114, w113) -> (w112:refnum<vi>[])
  n176 = while {
    stop <- FALSE stop-if-true
    n177 = global read "质控中断报警全局.vi" "CODMn中断报警"() -> (→"CODMn质控中断报警":bool)
    n178 = global read "质控中断报警全局.vi" "氨氮中断报警"() -> (→"氨氮质控中断报警":bool)
    n179 = global read "质控中断报警全局.vi" "总氮中断报警"() -> (→"总氮质控中断报警":bool)
    n180 = global read "质控中断报警全局.vi" "总磷中断报警"() -> (→"总磷质控中断报警":bool)
    n181 = Wait (ms)(milliseconds to wait=u32 100 ("等待时间（毫秒）")) -> ()  [unwired: 1 out]
    n182 = local read "COD状态"() -> (w410:u16)
    n183 = local read "总氮状态"() -> (w408:u16)
    n184 = local read "氨氮状态"() -> (w424:u16)
    n185 = local read "总磷状态"() -> (w415:u16)
    n186 = Not Equal To 0?(x=w408) -> (x != 0?=w407:bool)
    n187 = Not Equal To 0?(x=w424) -> (x != 0?=w423:bool)
    n188 = Not Equal To 0?(x=w415) -> (x != 0?=w417:bool)
    n189 = Not Equal To 0?(x=w410) -> (x != 0?=w414:bool)
    n190 = Select(t=T11."Disabled and Grayed Out" ("禁用"), s=w423, f=T11."Enabled") -> (s? t:f=w420:T11)
    n191 = Select(t=T11."Disabled and Grayed Out" ("禁用"), s=w417, f=T11."Enabled") -> (s? t:f=w416:T11)
    n192 = Select(t=T11."Disabled and Grayed Out" ("禁用"), s=w414, f=T11."Enabled") -> (s? t:f=w411:T11)
    n193 = Select(t=T11."Disabled and Grayed Out" ("禁用"), s=w407, f=T11."Enabled") -> (s? t:f=w404:T11)
    n194 = property on="氨氮调试" class="Bool"("DisabledEnum"=w420) -> ()  [unwired: 2 in, 2 out]
    n195 = property on="总磷调试" class="Bool"("DisabledEnum"=w416) -> ()  [unwired: 2 in, 2 out]
    n196 = property on="COD调试" class="Bool"("DisabledEnum"=w411) -> ()  [unwired: 2 in, 2 out]
    n197 = property on="总氮调试" class="Bool"("DisabledEnum"=w404) -> ()  [unwired: 2 in, 2 out]
    n198 = case shown="真" "启用" {
      frame False {
      }
      frame True {
        w442 = T12 0 items=["最小二乘", "最小绝对残差", "Bisquare"] ("method")
        n199 = Build Array("标准体积 1", "标准体积 2", "标准体积 3", "标准体积 4", "标准体积 5") -> (w439:dbl[])
        n200 = Build Array("实际体积 1", "实际体积 2", "实际体积 3", "实际体积 4", "实际体积 5") -> (w440:dbl[])
        n201 = call "线性公式质控用.vi"("标液浓度"=w439, "模型"=enum32{"线性", "多项式"}."线性", "监测浓度"=w440, "启用"=bool[] [TRUE, TRUE, TRUE, TRUE, TRUE], "method"=w442) -> ("拟合方程"=→"拟合方程":string, "r^2"=→"r^2":dbl, "slope"=w428:dbl, "intercept"=w427:dbl)  [unwired: 6 in, 1 out]
        n202 = case shown="\"柱塞泵3\"" "枚举" {
          tunnel: w428 -> [w446 w449 w450]
          tunnel: w427 -> [w447 w448 w451]
          frame "柱塞泵1", Default {
            n203 = local write "K"(w446) -> ()
            n204 = local write "B"(w447) -> ()
          }
          frame "柱塞泵2" {
            n205 = local write "K 2"(w449) -> ()
            n206 = local write "B 2"(w448) -> ()
          }
          frame "柱塞泵3" {
            n207 = local write "K 3"(w450) -> ()
            n208 = local write "B 3"(w451) -> ()
          }
        }
      }
    }
  }
  n209 = control-ref of="总磷加标水杯定容体积"() -> (w153:refnum<vi>)
  n210 = control-ref of="氨氮加标水杯定容体积"() -> (w195:refnum<vi>)
  n211 = Unbundle By Name(w188) -> ("量程"=→"氨氮量程":dbl, "检出限"=→"氨氮检出限":dbl, "加标前水样浓度"=→"氨氮加标前水样浓度":dbl, "加标后水样浓度"=→"氨氮加标后水样浓度":dbl, "加标水杯定容体积"=→"氨氮加标水杯定容体积":dbl, "加标母液浓度"=→"氨氮母液浓度":dbl, "加标体积"=→"氨氮加标体积":dbl, "加标回收率"=→"氨氮加标回收率":dbl)
  n212 = control-ref of="总磷加标前水样浓度"() -> (w155:refnum<vi>)
  n213 = control-ref of="总磷加标后水样浓度"() -> (w154:refnum<vi>)
  n214 = control-ref of="氨氮加标前水样浓度"() -> (w196:refnum<vi>)
  n215 = control-ref of="氨氮加标后水样浓度"() -> (w192:refnum<vi>)
  n216 = control-ref of="COD加标回收率"() -> (w141:refnum<vi>)
  n217 = control-ref of="COD母液浓度"() -> (w143:refnum<vi>)
  n218 = control-ref of="COD加标体积"() -> (w142:refnum<vi>)
  n219 = call "质控参数读取.vi"("section"="总磷质控参数", "error in (no error)"=w169) -> ("error out"=w166:errorcluster, "参数"=w178:T8)  [unwired: 8 in]
  n220 = control-ref of="总磷加标回收率"() -> (w151:refnum<vi>)
  n221 = control-ref of="氨氮加标回收率"() -> (w190:refnum<vi>)
  n222 = control-ref of="COD检出限"() -> (w147:refnum<vi>)
  n223 = control-ref of="总磷母液浓度"() -> (w152:refnum<vi>)
  n224 = control-ref of="总磷加标体积"() -> (w150:refnum<vi>)
  n225 = control-ref of="氨氮母液浓度"() -> (w194:refnum<vi>)
  n226 = control-ref of="氨氮加标体积"() -> (w191:refnum<vi>)
  n227 = control-ref of="COD量程"() -> (w148:refnum<vi>)
  n228 = control-ref of="总磷检出限"() -> (w156:refnum<vi>)
  n229 = control-ref of="氨氮检出限"() -> (w197:refnum<vi>)
  n230 = control-ref of="总磷量程"() -> (w157:refnum<vi>)
  n231 = control-ref of="氨氮量程"() -> (w198:refnum<vi>)
  n232 = Obtain Notifier(name (unnamed)="采配水Process" ("名称（未命名）"), notification data type=FALSE) -> (notifier out=w132:refnum<notifier>)  [unwired: 2 in, 2 out]
  n233 = Build Array(w148, w147, w146, w145, w144, w143, w142, w141) -> (w140:refnum<vi>[])
  n234 = Build Array(w157, w156, w155, w154, w153, w152, w150, w151) -> (w149:refnum<vi>[])
  n235 = Build Array(w198, w197, w196, w192, w195, w194, w191, w190) -> (w193:refnum<vi>[])
  n236 = Unbundle By Name(w178) -> ("量程"=→"总磷量程":dbl, "检出限"=→"总磷检出限":dbl, "加标前水样浓度"=→"总磷加标前水样浓度":dbl, "加标后水样浓度"=→"总磷加标后水样浓度":dbl, "加标水杯定容体积"=→"总磷加标水杯定容体积":dbl, "加标母液浓度"=→"总磷母液浓度":dbl, "加标体积"=→"总磷加标体积":dbl, "加标回收率"=→"总磷加标回收率":dbl)
  n237 = call "质控参数读取.vi"("section"="COD质控参数", "error in (no error)"=w166) -> ("error out"=w110:errorcluster, "参数"=w168:T8)  [unwired: 8 in]
  n238 = call "质控参数读取.vi"("section"="总氮质控参数", "error in (no error)"=w110) -> ("参数"=w109:T8)  [unwired: 8 in, 1 out]
  n239 = Unbundle By Name(w109) -> ("量程"=→"总氮量程":dbl, "检出限"=→"总氮检出限":dbl, "加标前水样浓度"=→"总氮加标前水样浓度":dbl, "加标后水样浓度"=→"总氮加标后水样浓度":dbl, "加标水杯定容体积"=→"总氮加标水杯定容体积":dbl, "加标母液浓度"=→"总氮母液浓度":dbl, "加标体积"=→"总氮加标体积":dbl, "加标回收率"=→"总氮加标回收率":dbl)
  n240 = Unbundle By Name(w168) -> ("量程"=→"COD量程":dbl, "检出限"=→"COD检出限":dbl, "加标前水样浓度"=→"COD加标前水样浓度":dbl, "加标后水样浓度"=→"COD加标后水样浓度":dbl, "加标水杯定容体积"=→"COD加标水杯定容体积":dbl, "加标母液浓度"=→"COD母液浓度":dbl, "加标体积"=→"COD加标体积":dbl, "加标回收率"=→"COD加标回收率":dbl)
  n241 = call <vilib>:"Application Directory.vi"() -> ("Application Directory"=w94:path)
  n242 = Build Path(base path=w94, name or relative path="data\\Set.ini" ("名称或相对路径")) -> (appended path=w92:path)
  n243 = call <vilib>:"Open Config Data.vi"("configuration file path"=w92) -> ("error out"=w90:errorcluster, "refnum"=w91:T13)  [unwired: 8 in, 1 out]
  n244 = call-poly <vilib>:"Read Key.vi"("section"=w88, "error in (no error)"=w90, "key"="背隙值1", "refnum"=w91) -> ("error out"=w85:errorcluster, "value"=w80:i32, "refnum out"=w87:T13)  [unwired: 4 in, 1 out]
  n245 = local write "背隙补偿步数"(w80) -> ()
  n246 = call-poly <vilib>:"Read Key.vi"("section"=w88, "error in (no error)"=w85, "key"="背隙值2", "refnum"=w87) -> ("error out"=w83:errorcluster, "value"=w81:i32, "refnum out"=w84:T13)  [unwired: 4 in, 1 out]
  n247 = Obtain Queue(name (unnamed)="采配水" ("名称（未命名）"), element data type=cluster{"命令":string, "数据":variant} {"命令"="", "数据"=variant}) -> (queue out=w122:refnum<queue>)  [unwired: 3 in, 2 out]
  n248 = while {
    tunnel: w193 -> [w457]
    tunnel: w149 -> [w456]
    tunnel: w140 -> [w455]
    tunnel: w132 -> [w454]
    tunnel: w122 -> [w453]
    tunnel: w112 -> [w452]
    stop <- FALSE stop-if-true
    # "氨氮站号是1，总磷总氮站号是2，COD站号是3"
    n249 = event shown="[41] \"报警清除\": 值改变" {
      selector: _ -> [_ _ _ _ _ _ _ _ _ _ _ _ _ _ _ _ _ _ _ _ _ _ _ _ _ _ _ _ _ _ _ _ _ _ _ _ _ _ _ _ _ _ _ _ _ _ _ _ _]
      dyn-events: _ -> [_ _ _ _ _ _ _ _ _ _ _ _ _ _ _ _ _ _ _ _ _ _ _ _ _ _ _ _ _ _ _ _ _ _ _ _ _ _ _ _ _ _ _ _ _ _ _ _ _]
      timeout: _ -> [_ _ _ _ _ _ _ _ _ _ _ _ _ _ _ _ _ _ _ _ _ _ _ _ _ _ _ _ _ _ _ _ _ _ _ _ _ _ _ _ _ _ _ _ _ _ _ _ _]
      tunnel: w457 -> [_ _ _ _ _ _ _ _ _ _ _ _ _ _ _ _ _ _ _ _ _ _ _ _ _ _ _ _ _ _ _ _ _ w777 _ _ _ w853 _ _ _ _ _ _ _ _ _ _ _]
      tunnel: w456 -> [_ _ _ _ _ _ _ _ _ _ _ _ _ _ _ _ _ _ _ _ _ _ _ _ _ _ _ _ _ _ _ _ _ _ w791 _ _ w850 _ _ _ _ _ _ _ _ _ _ _]
      tunnel: w455 -> [_ _ _ _ _ _ _ _ _ _ _ _ _ _ _ _ _ _ _ _ _ _ _ _ _ _ _ _ _ _ _ _ _ _ _ _ w829 w849 _ _ _ _ _ _ _ _ _ _ _]
      tunnel: w454 -> [_ _ _ _ _ _ _ _ _ _ _ _ _ _ _ _ _ _ _ _ _ _ _ _ _ _ _ _ _ _ _ _ _ _ _ _ _ _ _ _ w878 _ _ _ _ w1001 w1031 _ _]
      tunnel: w453 -> [_ _ _ _ _ _ _ _ _ _ _ _ _ _ _ _ _ _ _ _ _ _ _ _ _ _ _ _ _ _ _ _ _ _ _ _ _ _ _ _ _ _ _ _ _ _ w1028 _ _]
      tunnel: w452 -> [_ _ _ _ _ _ _ _ _ _ _ _ _ _ _ _ _ _ _ _ _ _ _ _ _ _ _ _ _ _ _ _ _ _ _ w809 _ _ _ _ _ _ _ _ _ _ _ _ _]
      tunnel: [_ _ _ _ _ _ _ _ _ _ _ _ _ _ _ _ _ _ _ _ _ _ _ _ _ _ _ _ _ w713 w750 w757 w764 _ _ _ _ _ _ _ _ w909 _ _ _ _ _ _ _] -> _
      event Timeout {
        n250 = event-data() -> ()  [unwired: 1 in, 3 out]
      }
      event "氨氮量程", "氨氮检出限", "氨氮加标前水样浓度", "氨氮加标水杯定容体积", "氨氮母液浓度", "氨氮加标后水样浓度": Mouse Down {
        n251 = event-data() -> ("CtlRef"=w462:refnum<vi>)  [unwired: 1 in, 7 out]
        n252 = property class="DigNum (严格)"(reference=w462) -> (reference out=w460:refnum<vi>, "Value"=w461:dbl)  [unwired: 1 in, 1 out]
        n253 = call "数字键盘.vi"("OldNumber"=w461) -> ("NewNumber"=w459:sgl)
        n254 = property class="DigNum (严格)"(reference=w460, "Val(Sgnl)"=w459) -> ()  [unwired: 1 in, 2 out]
      }
      event "总磷母液浓度", "总磷加标水杯定容体积", "总磷加标后水样浓度", "总磷加标前水样浓度", "总磷检出限", "总磷量程": Mouse Down {
        n255 = event-data() -> ("CtlRef"=w466:refnum<vi>)  [unwired: 1 in, 7 out]
        n256 = property class="DigNum (严格)"(reference=w466) -> (reference out=w464:refnum<vi>, "Value"=w465:dbl)  [unwired: 1 in, 1 out]
        n257 = call "数字键盘.vi"("OldNumber"=w465) -> ("NewNumber"=w463:sgl)
        n258 = property class="DigNum (严格)"(reference=w464, "Val(Sgnl)"=w463) -> ()  [unwired: 1 in, 2 out]
      }
      event "总氮母液浓度", "总氮加标水杯定容体积", "总氮加标后水样浓度", "总氮加标前水样浓度", "总氮检出限", "总氮量程": Mouse Down {
        n259 = event-data() -> ("CtlRef"=w470:refnum<vi>)  [unwired: 1 in, 7 out]
        n260 = property class="DigNum (严格)"(reference=w470) -> (reference out=w468:refnum<vi>, "Value"=w469:dbl)  [unwired: 1 in, 1 out]
        n261 = call "数字键盘.vi"("OldNumber"=w469) -> ("NewNumber"=w467:sgl)
        n262 = property class="DigNum (严格)"(reference=w468, "Val(Sgnl)"=w467) -> ()  [unwired: 1 in, 2 out]
      }
      event "COD母液浓度", "COD加标水杯定容体积", "COD加标后水样浓度", "COD加标前水样浓度", "COD检出限", "COD量程": Mouse Down {
        n263 = event-data() -> ("CtlRef"=w474:refnum<vi>)  [unwired: 1 in, 7 out]
        n264 = property class="DigNum (严格)"(reference=w474) -> (reference out=w472:refnum<vi>, "Value"=w473:dbl)  [unwired: 1 in, 1 out]
        n265 = call "数字键盘.vi"("OldNumber"=w473) -> ("NewNumber"=w471:sgl)
        n266 = property class="DigNum (严格)"(reference=w472, "Val(Sgnl)"=w471) -> ()  [unwired: 1 in, 2 out]
      }
      event "背隙补偿步数": Mouse Down {
        n267 = event-data() -> ()  [unwired: 1 in, 8 out]
        n268 = local read "背隙补偿步数"() -> (w476:i32)
        n269 = call "数字键盘.vi"("OldNumber"=w476) -> ("NewNumber"=w475:sgl)
        n270 = local write "背隙补偿步数"(w475) -> ()
      }
      event "标准体积 1": Mouse Down {
        n271 = event-data() -> ()  [unwired: 1 in, 8 out]
        n272 = local read "标准体积 1"() -> (w478:dbl)
        n273 = call "数字键盘.vi"("OldNumber"=w478) -> ("NewNumber"=w477:sgl)
        n274 = local write "标准体积 1"(w477) -> ()
      }
      event "标准体积 2": Mouse Down {
        n275 = event-data() -> ()  [unwired: 1 in, 8 out]
        n276 = local read "标准体积 2"() -> (w480:dbl)
        n277 = call "数字键盘.vi"("OldNumber"=w480) -> ("NewNumber"=w479:sgl)
        n278 = local write "标准体积 2"(w479) -> ()
      }
      event "标准体积 3": Mouse Down {
        n279 = event-data() -> ()  [unwired: 1 in, 8 out]
        n280 = local read "标准体积 3"() -> (w482:dbl)
        n281 = call "数字键盘.vi"("OldNumber"=w482) -> ("NewNumber"=w481:sgl)
        n282 = local write "标准体积 3"(w481) -> ()
      }
      event "标准体积 4": Mouse Down {
        n283 = event-data() -> ()  [unwired: 1 in, 8 out]
        n284 = local read "标准体积 4"() -> (w484:dbl)
        n285 = call "数字键盘.vi"("OldNumber"=w484) -> ("NewNumber"=w483:sgl)
        n286 = local write "标准体积 4"(w483) -> ()
      }
      event "标准体积 5": Mouse Down {
        n287 = event-data() -> ()  [unwired: 1 in, 8 out]
        n288 = local read "标准体积 5"() -> (w486:dbl)
        n289 = call "数字键盘.vi"("OldNumber"=w486) -> ("NewNumber"=w485:sgl)
        n290 = local write "标准体积 5"(w485) -> ()
      }
      event "实际体积 1": Mouse Down {
        n291 = event-data() -> ()  [unwired: 1 in, 8 out]
        n292 = local read "实际体积 1"() -> (w488:dbl)
        n293 = call "数字键盘.vi"("OldNumber"=w488) -> ("NewNumber"=w487:sgl)
        n294 = local write "实际体积 1"(w487) -> ()
      }
      event "实际体积 2": Mouse Down {
        n295 = event-data() -> ()  [unwired: 1 in, 8 out]
        n296 = local read "实际体积 2"() -> (w490:dbl)
        n297 = call "数字键盘.vi"("OldNumber"=w490) -> ("NewNumber"=w489:sgl)
        n298 = local write "实际体积 2"(w489) -> ()
      }
      event "实际体积 3": Mouse Down {
        n299 = event-data() -> ()  [unwired: 1 in, 8 out]
        n300 = local read "实际体积 3"() -> (w492:dbl)
        n301 = call "数字键盘.vi"("OldNumber"=w492) -> ("NewNumber"=w491:sgl)
        n302 = local write "实际体积 3"(w491) -> ()
      }
      event "实际体积 4": Mouse Down {
        n303 = event-data() -> ()  [unwired: 1 in, 8 out]
        n304 = local read "实际体积 4"() -> (w494:dbl)
        n305 = call "数字键盘.vi"("OldNumber"=w494) -> ("NewNumber"=w493:sgl)
        n306 = local write "实际体积 4"(w493) -> ()
      }
      event "实际体积 5": Mouse Down {
        n307 = event-data() -> ()  [unwired: 1 in, 8 out]
        n308 = local read "实际体积 5"() -> (w496:dbl)
        n309 = call "数字键盘.vi"("OldNumber"=w496) -> ("NewNumber"=w495:sgl)
        n310 = local write "实际体积 5"(w495) -> ()
      }
      event "K": Mouse Down {
        n311 = event-data() -> ()  [unwired: 1 in, 8 out]
        n312 = local read "K"() -> (w498:dbl)
        n313 = call "数字键盘.vi"("OldNumber"=w498) -> ("NewNumber"=w497:sgl)
        n314 = local write "K"(w497) -> ()
      }
      event "B": Mouse Down {
        n315 = event-data() -> ()  [unwired: 1 in, 8 out]
        n316 = local read "B"() -> (w500:dbl)
        n317 = call "数字键盘.vi"("OldNumber"=w500) -> ("NewNumber"=w499:sgl)
        n318 = local write "B"(w499) -> ()
      }
      event "K 2": Mouse Down {
        n319 = event-data() -> ()  [unwired: 1 in, 8 out]
        n320 = local read "K 2"() -> (w502:dbl)
        n321 = call "数字键盘.vi"("OldNumber"=w502) -> ("NewNumber"=w501:sgl)
        n322 = local write "K 2"(w501) -> ()
      }
      event "B 2": Mouse Down {
        n323 = event-data() -> ()  [unwired: 1 in, 8 out]
        n324 = local read "B 2"() -> (w504:dbl)
        n325 = call "数字键盘.vi"("OldNumber"=w504) -> ("NewNumber"=w503:sgl)
        n326 = local write "B 2"(w503) -> ()
      }
      event "K 3": Mouse Down {
        n327 = event-data() -> ()  [unwired: 1 in, 8 out]
        n328 = local read "K 3"() -> (w506:dbl)
        n329 = call "数字键盘.vi"("OldNumber"=w506) -> ("NewNumber"=w505:sgl)
        n330 = local write "K 3"(w505) -> ()
      }
      event "B 3": Mouse Down {
        n331 = event-data() -> ()  [unwired: 1 in, 8 out]
        n332 = local read "B 3"() -> (w508:dbl)
        n333 = call "数字键盘.vi"("OldNumber"=w508) -> ("NewNumber"=w507:sgl)
        n334 = local write "B 3"(w507) -> ()
      }
      event "背隙补偿步数 2": Mouse Down {
        n335 = event-data() -> ()  [unwired: 1 in, 8 out]
        n336 = local read "背隙补偿步数 2"() -> (w509:i32)
        n337 = call "数字键盘.vi"("OldNumber"=w509) -> ("NewNumber"=w510:sgl)
        n338 = local write "背隙补偿步数 2"(w510) -> ()
      }
      event "背隙补偿步数 3": Mouse Down {
        n339 = event-data() -> ()  [unwired: 1 in, 8 out]
        n340 = local read "背隙补偿步数 3"() -> (w512:i32)
        n341 = call "数字键盘.vi"("OldNumber"=w512) -> ("NewNumber"=w511:sgl)
        n342 = local write "背隙补偿步数 3"(w511) -> ()
      }
      event "背隙补偿步数", "背隙补偿步数 2", "背隙补偿步数 3", "标准体积 1", "标准体积 2", "标准体积 3", "标准体积 4", "标准体积 5", "实际体积 1", "实际体积 2", "实际体积 3", "实际体积 4", "实际体积 5": Value Change {
        w533 = "质控线性参数" ("section")
        w564 = "质控背隙补偿" ("section")
        n343 = event-data() -> ()  [unwired: 1 in, 6 out]
        n344 = call <vilib>:"Application Directory.vi"() -> ("Application Directory"=w571:path)
        n345 = Build Path(base path=w571, name or relative path="data\\Set.ini" ("名称或相对路径")) -> (appended path=w569:path)
        n346 = call <vilib>:"Open Config Data.vi"("configuration file path"=w569) -> ("error out"=w567:errorcluster, "refnum"=w568:T13)  [unwired: 8 in, 1 out]
        n347 = call-poly <vilib>:"Write Key.vi"("section"=w564, "error in (no error)"=w567, "value"="背隙补偿步数", "key"="背隙值1", "refnum"=w568) -> ("error out"=w558:errorcluster, "refnum out"=w561:T13)  [unwired: 4 in, 1 out]
        n348 = call-poly <vilib>:"Write Key.vi"("section"=w564, "error in (no error)"=w558, "value"="背隙补偿步数 2", "key"="背隙值2", "refnum"=w561) -> ("error out"=w559:errorcluster, "refnum out"=w560:T13)  [unwired: 4 in, 1 out]
        n349 = local read "标准体积 1"() -> (w531:dbl)
        n350 = call-poly <vilib>:"Write Key.vi"("section"=w564, "error in (no error)"=w559, "value"="背隙补偿步数 3", "key"="背隙值3", "refnum"=w560) -> ("error out"=w554:errorcluster, "refnum out"=w555:T13)  [unwired: 4 in, 1 out]
        n351 = local read "标准体积 2"() -> (w530:dbl)
        n352 = local read "标准体积 3"() -> (w528:dbl)
        n353 = call-poly <vilib>:"Write Key.vi"("section"=w533, "error in (no error)"=w554, "value"=w531, "key"="标准体积1", "refnum"=w555) -> ("error out"=w552:errorcluster, "refnum out"=w553:T13)  [unwired: 4 in, 1 out]
        n354 = local read "标准体积 4"() -> (w524:dbl)
        n355 = call-poly <vilib>:"Write Key.vi"("section"=w533, "error in (no error)"=w552, "value"=w530, "key"="标准体积2", "refnum"=w553) -> ("error out"=w550:errorcluster, "refnum out"=w551:T13)  [unwired: 4 in, 1 out]
        n356 = call-poly <vilib>:"Write Key.vi"("section"=w533, "error in (no error)"=w550, "value"=w528, "key"="标准体积3", "refnum"=w551) -> ("error out"=w548:errorcluster, "refnum out"=w549:T13)  [unwired: 4 in, 1 out]
        n357 = local read "标准体积 5"() -> (w523:dbl)
        n358 = call-poly <vilib>:"Write Key.vi"("section"=w533, "error in (no error)"=w548, "value"=w524, "key"="标准体积4", "refnum"=w549) -> ("error out"=w546:errorcluster, "refnum out"=w547:T13)  [unwired: 4 in, 1 out]
        n359 = local read "实际体积 1"() -> (w517:dbl)
        n360 = call-poly <vilib>:"Write Key.vi"("section"=w533, "error in (no error)"=w546, "value"=w523, "key"="标准体积5", "refnum"=w547) -> ("error out"=w544:errorcluster, "refnum out"=w545:T13)  [unwired: 4 in, 1 out]
        n361 = local read "实际体积 2"() -> (w516:dbl)
        n362 = call-poly <vilib>:"Write Key.vi"("section"=w533, "error in (no error)"=w544, "value"=w517, "key"="实际体积1", "refnum"=w545) -> ("error out"=w542:errorcluster, "refnum out"=w543:T13)  [unwired: 4 in, 1 out]
        n363 = local read "实际体积 3"() -> (w515:dbl)
        n364 = local read "实际体积 4"() -> (w514:dbl)
        n365 = call-poly <vilib>:"Write Key.vi"("section"=w533, "error in (no error)"=w542, "value"=w516, "key"="实际体积2", "refnum"=w543) -> ("error out"=w540:errorcluster, "refnum out"=w541:T13)  [unwired: 4 in, 1 out]
        n366 = local read "实际体积 5"() -> (w513:dbl)
        n367 = call-poly <vilib>:"Write Key.vi"("section"=w533, "error in (no error)"=w540, "value"=w515, "key"="实际体积3", "refnum"=w541) -> ("error out"=w538:errorcluster, "refnum out"=w539:T13)  [unwired: 4 in, 1 out]
        n368 = call-poly <vilib>:"Write Key.vi"("section"=w533, "error in (no error)"=w538, "value"=w514, "key"="实际体积4", "refnum"=w539) -> ("error out"=w536:errorcluster, "refnum out"=w537:T13)  [unwired: 4 in, 1 out]
        n369 = call-poly <vilib>:"Write Key.vi"("section"=w533, "error in (no error)"=w536, "value"=w513, "key"="实际体积5", "refnum"=w537) -> ("error out"=w534:errorcluster, "refnum out"=w535:T13)  [unwired: 4 in, 1 out]
        n370 = call <vilib>:"Close Config Data.vi"("error in (no error)"=w534, "refnum"=w535) -> ()  [unwired: 8 in, 2 out]
      }
      event "模块选择", "模块选择 2", "模块选择 3": Value Change {
        w586 = "质控模块选择" ("section")
        n371 = event-data() -> ()  [unwired: 1 in, 6 out]
        n372 = call <vilib>:"Application Directory.vi"() -> ("Application Directory"=w589:path)
        n373 = Build Path(base path=w589, name or relative path="data\\Set.ini" ("名称或相对路径")) -> (appended path=w587:path)
        n374 = local read "模块选择"() -> (w576:bool)
        n375 = call <vilib>:"Open Config Data.vi"("configuration file path"=w587) -> ("error out"=w584:errorcluster, "refnum"=w585:T13)  [unwired: 8 in, 1 out]
        n376 = local read "模块选择 2"() -> (w575:bool)
        n377 = call-poly <vilib>:"Write Key.vi"("section"=w586, "error in (no error)"=w584, "value"=w576, "key"="模块1" ("section"), "refnum"=w585) -> ("error out"=w582:errorcluster, "refnum out"=w583:T13)  [unwired: 4 in, 1 out]
        n378 = local read "模块选择 3"() -> (w574:bool)
        n379 = call-poly <vilib>:"Write Key.vi"("section"=w586, "error in (no error)"=w582, "value"=w575, "key"="模块2" ("section"), "refnum"=w583) -> ("error out"=w580:errorcluster, "refnum out"=w581:T13)  [unwired: 4 in, 1 out]
        n380 = call-poly <vilib>:"Write Key.vi"("section"=w586, "error in (no error)"=w580, "value"=w574, "key"="模块3" ("section"), "refnum"=w581) -> ("error out"=w572:errorcluster, "refnum out"=w573:T13)  [unwired: 4 in, 1 out]
        n381 = call <vilib>:"Close Config Data.vi"("error in (no error)"=w572, "refnum"=w573) -> ()  [unwired: 8 in, 2 out]
      }
      event "氨氮量程选择", "总氮量程选择", "总磷量程选择", "CODMn量程选择": Value Change {
        w594 = "质控模块量程选择" ("section")
        n382 = event-data() -> ()  [unwired: 1 in, 6 out]
        n383 = call <vilib>:"Application Directory.vi"() -> ("Application Directory"=w611:path)
        n384 = Build Path(base path=w611, name or relative path="data\\Set.ini" ("名称或相对路径")) -> (appended path=w609:path)
        n385 = local read "氨氮量程选择"() -> (w593:enum32{"H", "L", "AUTO"})
        n386 = call <vilib>:"Open Config Data.vi"("configuration file path"=w609) -> ("error out"=w607:errorcluster, "refnum"=w608:T13)  [unwired: 8 in, 1 out]
        n387 = local read "总氮量程选择"() -> (w592:enum32{"H", "L", "AUTO"})
        n388 = call-poly <vilib>:"Write Key.vi"("section"=w594, "error in (no error)"=w607, "value"=w593, "key"="氨氮" ("section"), "refnum"=w608) -> ("error out"=w605:errorcluster, "refnum out"=w606:T13)  [unwired: 4 in, 1 out]
        n389 = local read "总磷量程选择"() -> (w591:enum32{"H", "L", "AUTO"})
        n390 = call-poly <vilib>:"Write Key.vi"("section"=w594, "error in (no error)"=w605, "value"=w592, "key"="总氮" ("section"), "refnum"=w606) -> ("error out"=w603:errorcluster, "refnum out"=w604:T13)  [unwired: 4 in, 1 out]
        n391 = local read "CODMn量程选择"() -> (w590:enum32{"H", "L", "AUTO"})
        n392 = call-poly <vilib>:"Write Key.vi"("section"=w594, "error in (no error)"=w603, "value"=w591, "key"="总磷" ("section"), "refnum"=w604) -> ("error out"=w598:errorcluster, "refnum out"=w599:T13)  [unwired: 4 in, 1 out]
        n393 = call-poly <vilib>:"Write Key.vi"("section"=w594, "error in (no error)"=w598, "value"=w590, "key"="CODMn" ("section"), "refnum"=w599) -> ("error out"=w596:errorcluster, "refnum out"=w597:T13)  [unwired: 4 in, 1 out]
        n394 = call <vilib>:"Close Config Data.vi"("error in (no error)"=w596, "refnum"=w597) -> ()  [unwired: 8 in, 2 out]
      }
      event "写入": Value Change {
        n395 = event-data() -> ()  [unwired: 1 in, 6 out]
        n396 = local read "枚举"() -> (w613:enum16{"柱塞泵1", "柱塞泵2", "柱塞泵3"})
        n397 = case shown="\"柱塞泵3\"" w613 {
          tunnel: [w614 w626 w637] -> w612
          frame "柱塞泵1", Default {
            n398 = local read "K"() -> (w618:dbl)
            n399 = local read "B"() -> (w619:dbl)
            n400 = local read "背隙补偿步数"() -> (w615:i32)
            n401 = Build Array(w618, w619) -> (w620:dbl[])
            n402 = call "浮点转CDAB整形ZK.vi"("浮点数"=w620) -> ("CDAB整形输出"=w622:u16[])  [unwired: 10 in]
            n403 = Build Array(w615) -> (w621:i32[])
            n404 = Insert Into Array(array=w621, index=0 ("索引"), new element=w622) -> (w624:i32[])
            n405 = call "写入参数.vi"("values"=w624, "starting address"=u16 1, "Slave ID"=u8 1) -> ("error out"=w614:errorcluster)  [unwired: 8 in]
          }
          frame "柱塞泵2" {
            n406 = local read "背隙补偿步数 2"() -> (w628:i32)
            n407 = local read "K 2"() -> (w631:dbl)
            n408 = local read "B 2"() -> (w630:dbl)
            n409 = Build Array(w631, w630) -> (w632:dbl[])
            n410 = call "浮点转CDAB整形ZK.vi"("浮点数"=w632) -> ("CDAB整形输出"=w633:u16[])  [unwired: 10 in]
            n411 = Build Array(w628) -> (w627:i32[])
            n412 = Insert Into Array(array=w627, index=0 ("索引"), new element=w633) -> (w635:i32[])
            n413 = call "写入参数.vi"("values"=w635, "starting address"=u16 1, "Slave ID"=u8 2) -> ("error out"=w626:errorcluster)  [unwired: 8 in]
          }
          frame "柱塞泵3" {
            n414 = local read "背隙补偿步数 3"() -> (w639:i32)
            n415 = local read "K 3"() -> (w643:dbl)
            n416 = local read "B 3"() -> (w644:dbl)
            n417 = Build Array(w643, w644) -> (w645:dbl[])
            n418 = call "浮点转CDAB整形ZK.vi"("浮点数"=w645) -> ("CDAB整形输出"=w646:u16[])  [unwired: 10 in]
            n419 = Build Array(w639) -> (w641:i32[])
            n420 = Insert Into Array(array=w641, index=0 ("索引"), new element=w646) -> (w640:i32[])
            n421 = call "写入参数.vi"("values"=w640, "starting address"=u16 1, "Slave ID"=u8 3) -> ("error out"=w637:errorcluster)  [unwired: 8 in]
          }
        }
        n422 = case shown="无错误" w612 {
          frame No Error {
            n423 = One Button Dialog(message="写入成功" ("消息"), button name ("OK")="确定" ("按钮名称（“确定”）")) -> ()  [unwired: 1 out]
          }
          frame Error {
            n424 = One Button Dialog(message="写入失败" ("消息"), button name ("OK")="确定" ("按钮名称（“确定”）")) -> ()  [unwired: 1 out]
          }
        }
      }
      event "读取": Value Change {
        n425 = event-data() -> ()  [unwired: 1 in, 6 out]
        n426 = local read "模块选择"() -> (w651:bool)
        n427 = case shown="假" w651 {
          tunnel: [errorcluster {"status"=FALSE, "code"=0, "source"=""} ("error out") w673] -> w664
          tunnel: [w666 w670] -> w661
          tunnel: [w665 w669] -> w660
          frame False {
            n428 = local read "簇"() -> (w667:T1)
            n429 = Unbundle By Name(w667) -> ("K3"=w666:sgl, "B3"=w665:sgl)
          }
          frame True {
            n430 = call "读取参数.vi"("Slave ID"=u8 1, "starting address"=u16 1, "quantity"=u16 4) -> ("values"=w672:u16[], "error out"=w673:errorcluster)  [unwired: 6 in]
            n431 = call "浮点CDAB转换质控.vi"("数组"=w672) -> ("数组 2"=w671:sgl[])  [unwired: 10 in]
            n432 = Index Array(array=w671) -> (element #1=w670:sgl, element #2=w669:sgl)  [unwired: 2 in]
          }
        }
        n433 = local read "模块选择 2"() -> (w652:bool)
        n434 = case shown="假" w652 {
          tunnel: w664 -> [w677 w688]
          tunnel: [w677 w687] -> w663
          tunnel: [w679 w684] -> w659
          tunnel: [w678 w683] -> w658
          frame False {
            n435 = local read "簇"() -> (w680:T1)
            n436 = Unbundle By Name(w680) -> ("K3"=w679:sgl, "B3"=w678:sgl)
          }
          frame True {
            n437 = call "读取参数.vi"("Slave ID"=u8 2, "starting address"=u16 1, "quantity"=u16 4, "Error in"=w688) -> ("values"=w686:u16[], "error out"=w687:errorcluster)  [unwired: 5 in]
            n438 = call "浮点CDAB转换质控.vi"("数组"=w686) -> ("数组 2"=w685:sgl[])  [unwired: 10 in]
            n439 = Index Array(array=w685) -> (element #1=w684:sgl, element #2=w683:sgl)  [unwired: 2 in]
          }
        }
        n440 = local read "模块选择 3"() -> (w653:bool)
        n441 = case shown="假" w653 {
          tunnel: w663 -> [w690 w701]
          tunnel: [w692 w698] -> w657
          tunnel: [w691 w697] -> w656
          tunnel: [w690 w694] -> w654
          frame False {
            n442 = local read "簇"() -> (w693:T1)
            n443 = Unbundle By Name(w693) -> ("K3"=w692:sgl, "B3"=w691:sgl)
          }
          frame True {
            n444 = call "读取参数.vi"("Slave ID"=u8 3, "starting address"=u16 1, "quantity"=u16 4, "Error in"=w701) -> ("values"=w700:u16[], "error out"=w694:errorcluster)  [unwired: 5 in]
            n445 = call "浮点CDAB转换质控.vi"("数组"=w700) -> ("数组 2"=w699:sgl[])  [unwired: 10 in]
            n446 = Index Array(array=w699) -> (element #1=w698:sgl, element #2=w697:sgl)  [unwired: 2 in]
          }
        }
        n447 = Bundle By Name(cluster=T1 {"K1"=0.0, "B1"=0.0, "K2"=0.0, "B2"=0.0, "K3"=0.0, "B3"=0.0} ("簇"), "K1"=w661, "B1"=w660, "K2"=w659, "B2"=w658, "K3"=w657, "B3"=w656) -> (→"簇":T1)
        n448 = case shown="无错误" w654 {
          frame No Error {
            n449 = One Button Dialog(message="读取成功" ("消息"), button name ("OK")="确定" ("按钮名称（“确定”）")) -> ()  [unwired: 1 out]
          }
          frame Error {
            n450 = One Button Dialog(message="读取失败" ("消息"), button name ("OK")="确定" ("按钮名称（“确定”）")) -> ()  [unwired: 1 out]
          }
        }
      }
      event "注出体积选择": Value Change {
        n451 = event-data() -> ()  [unwired: 1 in, 6 out]
        n452 = case shown="0" "注出体积选择" {
          tunnel: [0.1 0.3 0.5 0.8 1.0] -> w724
          frame 0 {
          }
          frame 1 {
          }
          frame 2 {
          }
          frame 3 {
          }
          frame 4, Default {
          }
        }
        n453 = local read "模块选择"() -> (w709:bool)
        n454 = Build Array(w724) -> (w711:dbl[])
        n455 = call "浮点转CDAB整形ZK.vi"("浮点数"=w711) -> ("CDAB整形输出"=w710:u16[])  [unwired: 10 in]
        n456 = case shown="假" w709 {
          tunnel: [_ w731] -> w727
          tunnel: [u16 8 ("starting address") w730] -> w725
          tunnel: w710 -> [_ w729]
          frame False {
          }
          frame True {
            w730 = u16 8 ("starting address")
            n457 = call "写入参数.vi"("values"=w729, "starting address"=w730, "Slave ID"=u8 1) -> ("error out"=w731:errorcluster)  [unwired: 8 in]
          }
        }
        n458 = local read "模块选择 2"() -> (w708:bool)
        n459 = case shown="真" w708 {
          tunnel: w727 -> [w733 w737]
          tunnel: [w733 w736] -> w726
          tunnel: w725 -> [_ w735]
          tunnel: w710 -> [_ w734]
          frame False {
          }
          frame True {
            n460 = call "写入参数.vi"("Error in"=w737, "values"=w734, "starting address"=w735, "Slave ID"=u8 2) -> ("error out"=w736:errorcluster)  [unwired: 7 in]
          }
        }
        n461 = local read "模块选择 3"() -> (w707:bool)
        n462 = case shown="真" w707 {
          tunnel: w726 -> [w739 w743]
          tunnel: w725 -> [_ w742]
          tunnel: [w739 w741] -> w720
          tunnel: w710 -> [_ w740]
          frame False {
          }
          frame True {
            n463 = call "写入参数.vi"("Error in"=w743, "values"=w740, "starting address"=w742, "Slave ID"=u8 3) -> ("error out"=w741:errorcluster)  [unwired: 7 in]
          }
        }
        n464 = call <vilib>:"Application Directory.vi"() -> ("Application Directory"=w723:path)
        n465 = Build Path(base path=w723, name or relative path="data\\Set.ini" ("名称或相对路径")) -> (appended path=w721:path)
        n466 = call <vilib>:"Open Config Data.vi"("error in (no error)"=w720, "configuration file path"=w721) -> ("error out"=w716:errorcluster, "refnum"=w717:T13)  [unwired: 7 in, 1 out]
        n467 = call-poly <vilib>:"Write Key.vi"("section"="质控手动体积选择", "error in (no error)"=w716, "value"="注出体积选择", "key"="手动体积选择" ("section"), "refnum"=w717) -> ("error out"=w718:errorcluster, "refnum out"=w719:T13)  [unwired: 4 in, 1 out]
        n468 = call <vilib>:"Close Config Data.vi"("error in (no error)"=w718, "refnum"=w719) -> ("error out"=w713:errorcluster)  [unwired: 8 in, 1 out]
      }
      event "柱塞泵1": Value Change {
        n469 = event-data() -> ()  [unwired: 1 in, 6 out]
        n470 = Build Array("柱塞泵1") -> (w751:bool[])
        n471 = call "多个线圈写入.vi"("values"=w751, "starting address"=u16 2104, "Slave ID"=u8 1) -> ("error out"=w750:errorcluster)  [unwired: 8 in]
        n472 = case shown="错误" w750 {
          frame No Error {
          }
          frame Error {
            n473 = One Button Dialog(message="启动失败" ("消息"), button name ("OK")="确定" ("按钮名称（“确定”）")) -> ()  [unwired: 1 out]
          }
        }
      }
      event "柱塞泵2": Value Change {
        n474 = event-data() -> ()  [unwired: 1 in, 6 out]
        n475 = Build Array("柱塞泵2") -> (w759:bool[])
        n476 = call "多个线圈写入.vi"("values"=w759, "starting address"=u16 2104, "Slave ID"=u8 2) -> ("error out"=w757:errorcluster)  [unwired: 8 in]
        n477 = case shown="错误" w757 {
          frame No Error {
          }
          frame Error {
            n478 = One Button Dialog(message="启动失败" ("消息"), button name ("OK")="确定" ("按钮名称（“确定”）")) -> ()  [unwired: 1 out]
          }
        }
      }
      event "柱塞泵3": Value Change {
        n479 = event-data() -> ()  [unwired: 1 in, 6 out]
        n480 = Build Array("柱塞泵3") -> (w766:bool[])
        n481 = call "多个线圈写入.vi"("values"=w766, "starting address"=u16 2104, "Slave ID"=u8 3) -> ("error out"=w764:errorcluster)  [unwired: 8 in]
        n482 = case shown="无错误" w764 {
          frame No Error {
          }
          frame Error {
            n483 = One Button Dialog(message="启动失败" ("消息"), button name ("OK")="确定" ("按钮名称（“确定”）")) -> ()  [unwired: 1 out]
          }
        }
      }
      event "氨氮量程", "氨氮检出限", "氨氮加标前水样浓度", "氨氮母液浓度", "氨氮加标水杯定容体积", "氨氮加标后水样浓度": Value Change {
        n484 = event-data() -> ()  [unwired: 1 in, 6 out]
        n485 = for {
          tunnel: w777 -> [w789] mode=indexing
          tunnel: [w788] -> w786 mode=indexing
          n486 = property class="DigNum (严格)"(reference=w789) -> ("Value"=w788:dbl)  [unwired: 1 in, 2 out]
        }
        n487 = Index Array(array=w786) -> (element #1=w785:dbl, element #2=w784:dbl, element #3=w771:dbl, element #4=w783:dbl, element #5=w782:dbl, element #6=w780:dbl)  [unwired: 6 in]
        n488 = Bundle By Name(cluster=T8 {"量程"=0.0, "检出限"=0.0, "加标前水样浓度"=0.0, "加标后水样浓度"=0.0, "加标水杯定容体积"=0.0, "加标母液浓度"=0.0, "加标体积"=0.0, "加标回收率"=0.0} ("参数"), "量程"=w785, "检出限"=w784, "加标前水样浓度"=w771, "加标后水样浓度"=w783, "加标水杯定容体积"=w782, "加标母液浓度"=w780) -> (w779:T8)
        n489 = global write "水样浓度全局.vi" "氨氮加标前水样浓度"(w771) -> ()
        n490 = call "加标回收率计算.vi"("参数"=w779) -> ("参数 out"=w778:T8)  [unwired: 10 in]
        n491 = Index Array(array=w777, index #1=6 ("索引")) -> (element #1=w776:refnum<vi>, element #2=w774:refnum<vi>)  [unwired: 1 in]
        n492 = call "质控参数保存.vi"("section"="氨氮质控参数", "参数"=w778) -> ()  [unwired: 9 in, 1 out]
        n493 = Unbundle By Name(w778) -> ("加标体积"=w772:dbl, "加标回收率"=w773:dbl)
        n494 = property class="DigNum (严格)"(reference=w776, "Value"=w772) -> ()  [unwired: 1 in, 2 out]
        n495 = property class="DigNum (严格)"(reference=w774, "Value"=w773) -> ()  [unwired: 1 in, 2 out]
      }
      event "总磷母液浓度", "总磷加标水杯定容体积", "总磷加标后水样浓度", "总磷加标前水样浓度", "总磷检出限", "总磷量程": Value Change {
        n496 = event-data() -> ()  [unwired: 1 in, 6 out]
        n497 = for {
          tunnel: w791 -> [w808] mode=indexing
          tunnel: [w807] -> w805 mode=indexing
          n498 = property class="DigNum (严格)"(reference=w808) -> ("Value"=w807:dbl)  [unwired: 1 in, 2 out]
        }
        n499 = Index Array(array=w805) -> (element #1=w804:dbl, element #2=w803:dbl, element #3=w790:dbl, element #4=w802:dbl, element #5=w801:dbl, element #6=w799:dbl)  [unwired: 6 in]
        n500 = global write "水样浓度全局.vi" "总磷加标前水样浓度"(w790) -> ()
        n501 = Bundle By Name(cluster=T8 {"量程"=0.0, "检出限"=0.0, "加标前水样浓度"=0.0, "加标后水样浓度"=0.0, "加标水杯定容体积"=0.0, "加标母液浓度"=0.0, "加标体积"=0.0, "加标回收率"=0.0} ("参数"), "量程"=w804, "检出限"=w803, "加标前水样浓度"=w790, "加标后水样浓度"=w802, "加标水杯定容体积"=w801, "加标母液浓度"=w799) -> (w798:T8)
        n502 = call "加标回收率计算.vi"("参数"=w798) -> ("参数 out"=w797:T8)  [unwired: 10 in]
        n503 = Index Array(array=w791, index #1=6 ("索引")) -> (element #1=w796:refnum<vi>, element #2=w793:refnum<vi>)  [unwired: 1 in]
        n504 = call "质控参数保存.vi"("section"="总磷质控参数", "参数"=w797) -> ()  [unwired: 9 in, 1 out]
        n505 = Unbundle By Name(w797) -> ("加标体积"=w794:dbl, "加标回收率"=w792:dbl)
        n506 = property class="DigNum (严格)"(reference=w796, "Value"=w794) -> ()  [unwired: 1 in, 2 out]
        n507 = property class="DigNum (严格)"(reference=w793, "Value"=w792) -> ()  [unwired: 1 in, 2 out]
      }
      event "总氮量程", "总氮检出限", "总氮加标前水样浓度", "总氮加标后水样浓度", "总氮加标水杯定容体积", "总氮母液浓度": Value Change {
        n508 = event-data() -> ()  [unwired: 1 in, 6 out]
        n509 = for {
          tunnel: w809 -> [w827] mode=indexing
          tunnel: [w826] -> w824 mode=indexing
          n510 = property class="DigNum (严格)"(reference=w827) -> ("Value"=w826:dbl)  [unwired: 1 in, 2 out]
        }
        n511 = Index Array(array=w824) -> (element #1=w823:dbl, element #2=w822:dbl, element #3=w810:dbl, element #4=w821:dbl, element #5=w820:dbl, element #6=w818:dbl)  [unwired: 6 in]
        n512 = global write "水样浓度全局.vi" "总氮加标前水样浓度"(w810) -> ()
        n513 = Bundle By Name(cluster=T8 {"量程"=0.0, "检出限"=0.0, "加标前水样浓度"=0.0, "加标后水样浓度"=0.0, "加标水杯定容体积"=0.0, "加标母液浓度"=0.0, "加标体积"=0.0, "加标回收率"=0.0} ("参数"), "量程"=w823, "检出限"=w822, "加标前水样浓度"=w810, "加标后水样浓度"=w821, "加标水杯定容体积"=w820, "加标母液浓度"=w818) -> (w817:T8)
        n514 = call "加标回收率计算.vi"("参数"=w817) -> ("参数 out"=w816:T8)  [unwired: 10 in]
        n515 = Index Array(array=w809, index #1=6 ("索引")) -> (element #1=w815:refnum<vi>, element #2=w812:refnum<vi>)  [unwired: 1 in]
        n516 = call "质控参数保存.vi"("section"="总氮质控参数", "参数"=w816) -> ()  [unwired: 9 in, 1 out]
        n517 = Unbundle By Name(w816) -> ("加标体积"=w813:dbl, "加标回收率"=w811:dbl)
        n518 = property class="DigNum (严格)"(reference=w815, "Value"=w813) -> ()  [unwired: 1 in, 2 out]
        n519 = property class="DigNum (严格)"(reference=w812, "Value"=w811) -> ()  [unwired: 1 in, 2 out]
      }
      event "COD母液浓度", "COD加标水杯定容体积", "COD加标后水样浓度", "COD加标前水样浓度", "COD检出限", "COD量程": Value Change {
        n520 = event-data() -> ()  [unwired: 1 in, 6 out]
        n521 = for {
          tunnel: w829 -> [w846] mode=indexing
          tunnel: [w845] -> w843 mode=indexing
          n522 = property class="DigNum (严格)"(reference=w846) -> ("Value"=w845:dbl)  [unwired: 1 in, 2 out]
        }
        n523 = Index Array(array=w843) -> (element #1=w842:dbl, element #2=w841:dbl, element #3=w828:dbl, element #4=w840:dbl, element #5=w839:dbl, element #6=w837:dbl)  [unwired: 6 in]
        n524 = global write "水样浓度全局.vi" "COD加标前水样浓度"(w828) -> ()
        n525 = Bundle By Name(cluster=T8 {"量程"=0.0, "检出限"=0.0, "加标前水样浓度"=0.0, "加标后水样浓度"=0.0, "加标水杯定容体积"=0.0, "加标母液浓度"=0.0, "加标体积"=0.0, "加标回收率"=0.0} ("参数"), "量程"=w842, "检出限"=w841, "加标前水样浓度"=w828, "加标后水样浓度"=w840, "加标水杯定容体积"=w839, "加标母液浓度"=w837) -> (w836:T8)
        n526 = call "加标回收率计算.vi"("参数"=w836) -> ("参数 out"=w835:T8)  [unwired: 10 in]
        n527 = Index Array(array=w829, index #1=6 ("索引")) -> (element #1=w834:refnum<vi>, element #2=w831:refnum<vi>)  [unwired: 1 in]
        n528 = call "质控参数保存.vi"("section"="COD质控参数", "参数"=w835) -> ()  [unwired: 9 in, 1 out]
        n529 = Unbundle By Name(w835) -> ("加标体积"=w832:dbl, "加标回收率"=w830:dbl)
        n530 = property class="DigNum (严格)"(reference=w834, "Value"=w832) -> ()  [unwired: 1 in, 2 out]
        n531 = property class="DigNum (严格)"(reference=w831, "Value"=w830) -> ()  [unwired: 1 in, 2 out]
      }
      event "氨氮调试", "总磷调试", "CODMn调试", "总氮调试": Value Change {
        n532 = event-data() -> ("CtlRef"=w852:refnum<vi>)  [unwired: 1 in, 5 out]
        n533 = property class="Bool"(reference=w852) -> ("Label.Text"=w851:string)  [unwired: 1 in, 2 out]
        n534 = case shown="\"CODMn调试\"" w851 {
          tunnel: w853 -> [w854 _ _ _]
          tunnel: w850 -> [_ w856 w858 _]
          tunnel: w849 -> [_ _ _ w860]
          tunnel: ["氨氮模块" ("标题") "总磷模块" ("标题") "总氮模块" ("标题") "CODMn模块" ("标题")] -> w848
          tunnel: [w854 w856 w858 w860] -> w847
          frame "氨氮调试", Default {
          }
          frame "总磷调试" {
          }
          frame "总氮调试" {
          }
          frame "CODMn调试" {
          }
        }
        n535 = call "加标模块单控对话框.vi"("数组"=w847, "标题"=w848) -> ()  [unwired: 10 in]
      }
      event "氨氮停止", "总磷停止", "CODMn停止", "总氮停止": Value Change {
        n536 = event-data() -> ("CtlRef"=w866:refnum<vi>)  [unwired: 1 in, 5 out]
        n537 = property class="Bool"(reference=w866) -> ("Label.Text"=w865:string)  [unwired: 1 in, 2 out]
        n538 = case shown="\"总氮停止\", \"总磷停止\"" w865 {
          tunnel: [u8 1 ("Slave ID") u8 2 ("Slave ID") u8 3 ("Slave ID")] -> w862
          frame "氨氮停止", Default {
          }
          frame "总氮停止", "总磷停止" {
          }
          frame "CODMn停止" {
          }
        }
        n539 = call "单个写入.vi"("value"=u16 2, "address"=u16 103, "Slave ID"=w862) -> ()  [unwired: 8 in, 1 out]
      }
      event "氨氮排液", "CODMn排液", "总磷排液", "总氮排液": Value Change {
        n540 = event-data() -> ("CtlRef"=w874:refnum<vi>)  [unwired: 1 in, 5 out]
        n541 = property class="Bool"(reference=w874) -> ("Label.Text"=w873:string)  [unwired: 1 in, 2 out]
        n542 = case shown="\"CODMn排液\"" w873 {
          tunnel: [u8 1 ("Slave ID") u8 2 ("Slave ID") u8 3 ("Slave ID")] -> w870
          frame "氨氮排液", Default {
          }
          frame "总氮排液", "总磷排液" {
          }
          frame "CODMn排液" {
          }
        }
        n543 = call "单个写入.vi"("value"=u16 3, "address"=u16 103, "Slave ID"=w870) -> ()  [unwired: 8 in, 1 out]
      }
      event "加标回收": Value Change {
        n544 = event-data() -> ()  [unwired: 1 in, 6 out]
        n545 = flat-sequence {
          tunnel: [w882] -> w881
          tunnel: [w886] -> w880
          tunnel: [w885] -> w879
          tunnel: w878 -> [w883]
          tunnel: w881 -> [w894]
          tunnel: w880 -> [w893]
          tunnel: w879 -> [w892]
          frame #0 {
            n546 = Send Notification(notification=FALSE ("通知"), notifier=w883) -> ()  [unwired: 1 in, 2 out]
            n547 = call "质控启动流程对话框.vi"() -> ("启动模块"=w882:T3, "直接启动"=w885:bool, "常规启动"=w886:bool)  [unwired: 8 in, 1 out]
            "常规启动" <- w886
            "直接启动" <- w885
            "启动模块" <- w882
          }
          frame #1 {
            n548 = Bundle By Name(cluster=T6 {"是否启用仪器"=FALSE, "CODMn"={"启动测量模式"={"测量模式"=enum."水样测量"}, "确定按钮"=FALSE}, "启动模块 3"={"氨氮"=FALSE, "总磷"=FALSE, "总氮"=FALSE, "COD"=FALSE}, "常规启动"=FALSE, "直接启动"=FALSE} ("输出簇"), "是否启用仪器"=TRUE, "启动模块 3"=w894, "常规启动"=w893, "直接启动"=w892) -> (w887:T6)
            "输出簇" <- w887
            n549 = vi-ref "质控单元.lvlib:古田户外一体站流程质控自动启动.vi"() -> (w890:refnum<vi>)
            n550 = property class="VI"(reference=w890) -> ("Name"=w891:string, "Exec.State"=w889:T15)  [unwired: 1 in, 2 out]
            n551 = case shown="\"Idle\"" w889 {
              tunnel: w891 -> [_ w906]
              tunnel: w887 -> [_ w905]
              frame "Bad", Default {
              }
              frame "Idle" {
                n552 = Open VI Reference(type specifier VI Refnum (for type only)=refnum<vi> refnum ("类型说明符VI引用句柄（仅用于类型）"), vi path=w906, options=128 ("选项")) -> (vi reference=w907:refnum<vi>, error out=w902:errorcluster)  [unwired: 3 in]
                n553 = call-by-ref "开始异步调用"(reference=w907, error in=w902, "CODMn量程切换"="CODMn量程选择", "总磷量程切换"="总磷量程选择", "总氮量程切换"="总氮量程选择", "氨氮量程切换"="氨氮量程选择", "参数"=w905) -> (reference out=w904:refnum<vi>, error out=w903:errorcluster)  [unwired: 7 in]
                n554 = Close Reference(reference=w904, error in (no error)=w903) -> ()  [unwired: 1 out]
              }
            }
          }
        }
      }
      event "报警清除": Value Change {
        w908 = FALSE ("氨氮中断报警")
        n555 = event-data() -> ()  [unwired: 1 in, 6 out]
        n556 = local read "模块选择"() -> (w920:bool)
        n557 = local read "模块选择"() -> (w911:bool)
        n558 = case shown="真" w920 {
          tunnel: [errorcluster {"status"=FALSE, "code"=0, "source"=""} ("error out") w951] -> w917
          frame False {
          }
          frame True {
            n559 = call "多个线圈写入.vi"("values"=bool[] [TRUE], "starting address"=u16 2106, "Slave ID"=u8 1) -> ("error out"=w951:errorcluster)  [unwired: 8 in]
          }
        }
        n560 = local read "模块选择 2"() -> (w919:bool)
        n561 = local read "模块选择 2"() -> (w912:bool)
        n562 = case shown="真" w919 {
          tunnel: w917 -> [w944 w947]
          tunnel: [w944 w945] -> w916
          frame False {
          }
          frame True {
            n563 = call "多个线圈写入.vi"("Error in"=w947, "values"=bool[] [TRUE], "starting address"=u16 2106, "Slave ID"=u8 2) -> ("error out"=w945:errorcluster)  [unwired: 7 in]
          }
        }
        n564 = local read "模块选择 3"() -> (w918:bool)
        n565 = local read "模块选择 3"() -> (w913:bool)
        n566 = global write "质控中断报警全局.vi" "CODMn中断报警"(w908) -> ()
        n567 = global write "质控中断报警全局.vi" "氨氮中断报警"(w908) -> ()
        n568 = global write "质控中断报警全局.vi" "总氮中断报警"(w908) -> ()
        n569 = global write "质控中断报警全局.vi" "总磷中断报警"(w908) -> ()
        n570 = case shown="真" w918 {
          tunnel: w916 -> [w938 w942]
          tunnel: [w938 w939] -> w910
          frame False {
          }
          frame True {
            n571 = call "多个线圈写入.vi"("Error in"=w942, "values"=bool[] [TRUE], "starting address"=u16 2106, "Slave ID"=u8 3) -> ("error out"=w939:errorcluster)  [unwired: 7 in]
          }
        }
        n572 = case shown="真" w911 {
          tunnel: [w933 w934] -> w914
          tunnel: w910 -> [w933 _]
          frame False {
          }
          frame True {
            n573 = call "多个线圈写入.vi"("values"=bool[] [FALSE], "starting address"=u16 2106, "Slave ID"=u8 1) -> ("error out"=w934:errorcluster)  [unwired: 8 in]
          }
        }
        n574 = case shown="真" w912 {
          tunnel: w914 -> [w927 w930]
          tunnel: [w927 w928] -> w915
          frame False {
          }
          frame True {
            n575 = call "多个线圈写入.vi"("Error in"=w930, "values"=bool[] [FALSE], "starting address"=u16 2106, "Slave ID"=u8 2) -> ("error out"=w928:errorcluster)  [unwired: 7 in]
          }
        }
        n576 = case shown="真" w913 {
          tunnel: w915 -> [w921 w925]
          tunnel: [w921 w922] -> w909
          frame False {
          }
          frame True {
            n577 = call "多个线圈写入.vi"("Error in"=w925, "values"=bool[] [FALSE], "starting address"=u16 2106, "Slave ID"=u8 3) -> ("error out"=w922:errorcluster)  [unwired: 7 in]
          }
        }
      }
      event "氨氮加标回收启动": Value Change {
        n578 = event-data() -> ()  [unwired: 1 in, 6 out]
        n579 = Two Button Dialog(message="确定启动氨氮的加标回收？" ("消息"), 1:"否" ("F按钮名称（“取消”）"), 2:"是" ("T按钮名称（“确定”）")) -> (T button?=w955:bool)
        n580 = case shown="真" w955 {
          frame False {
          }
          frame True {
            n581 = vi-ref "质控单元.lvlib:氨氮流程质控自动启动.vi"() -> (w961:refnum<vi>)
            n582 = property class="VI"(reference=w961) -> ("Name"=w959:string, "Exec.State"=w960:T15)  [unwired: 1 in, 2 out]
            n583 = case shown="\"Idle\"" w960 {
              tunnel: w959 -> [_ w965 _ _]
              frame "Bad", Default {
              }
              frame "Idle" {
                n584 = local read "氨氮量程选择"() -> (w964:enum32{"H", "L", "AUTO"})
                n585 = Open VI Reference(type specifier VI Refnum (for type only)=refnum<vi> refnum ("类型说明符VI引用句柄（仅用于类型）"), vi path=w965, options=128 ("选项")) -> (vi reference=w969:refnum<vi>, error out=w963:errorcluster)  [unwired: 3 in]
                n586 = call-by-ref "开始异步调用"(reference=w969, error in=w963, "氨氮量程切换"=w964) -> (reference out=w968:refnum<vi>, error out=w962:errorcluster)  [unwired: 11 in]
                n587 = Close Reference(reference=w968, error in (no error)=w962) -> ()  [unwired: 1 out]
              }
              frame "Run top level" {
              }
              frame "Running" {
              }
            }
          }
        }
      }
      event "总磷总氮加标回收启动": Value Change {
        n588 = event-data() -> ()  [unwired: 1 in, 6 out]
        n589 = Two Button Dialog(message="确定启动总磷总氮的加标回收？" ("消息"), 1:"否" ("F按钮名称（“取消”）"), 2:"是" ("T按钮名称（“确定”）")) -> (T button?=w970:bool)
        n590 = case shown="真" w970 {
          frame False {
          }
          frame True {
            n591 = vi-ref "质控单元.lvlib:总磷总氮流程质控自动启动.vi"() -> (w976:refnum<vi>)
            n592 = property class="VI"(reference=w976) -> ("Name"=w974:string, "Exec.State"=w975:T15)  [unwired: 1 in, 2 out]
            n593 = case shown="\"Idle\"" w975 {
              tunnel: w974 -> [_ w981 _ _]
              frame "Bad", Default {
              }
              frame "Idle" {
                n594 = local read "总氮量程选择"() -> (w978:enum32{"H", "L", "AUTO"})
                n595 = local read "总磷量程选择"() -> (w977:enum32{"H", "L", "AUTO"})
                n596 = Open VI Reference(type specifier VI Refnum (for type only)=refnum<vi> refnum ("类型说明符VI引用句柄（仅用于类型）"), vi path=w981, options=128 ("选项")) -> (vi reference=w985:refnum<vi>, error out=w979:errorcluster)  [unwired: 3 in]
                n597 = call-by-ref "开始异步调用"(reference=w985, error in=w979, "总磷量程切换"=w977, "总氮量程切换"=w978) -> (reference out=w984:refnum<vi>, error out=w980:errorcluster)  [unwired: 10 in]
                n598 = Close Reference(reference=w984, error in (no error)=w980) -> ()  [unwired: 1 out]
              }
              frame "Run top level" {
              }
              frame "Running" {
              }
            }
          }
        }
      }
      event "CODMn加标回收启动": Value Change {
        n599 = event-data() -> ()  [unwired: 1 in, 6 out]
        n600 = Two Button Dialog(message="确定启动CODMn的加标回收？" ("消息"), 1:"否" ("F按钮名称（“取消”）"), 2:"是" ("T按钮名称（“确定”）")) -> (T button?=w986:bool)
        n601 = case shown="真" w986 {
          frame False {
          }
          frame True {
            n602 = vi-ref "质控单元.lvlib:CODMn流程质控自动启动.vi"() -> (w992:refnum<vi>)
            n603 = property class="VI"(reference=w992) -> ("Name"=w990:string, "Exec.State"=w991:T15)  [unwired: 1 in, 2 out]
            n604 = case shown="\"Idle\"" w991 {
              tunnel: w990 -> [_ w996 _ _]
              frame "Bad", Default {
              }
              frame "Idle" {
                n605 = local read "CODMn量程选择"() -> (w993:enum32{"H", "L", "AUTO"})
                n606 = Open VI Reference(type specifier VI Refnum (for type only)=refnum<vi> refnum ("类型说明符VI引用句柄（仅用于类型）"), vi path=w996, options=128 ("选项")) -> (vi reference=w1000:refnum<vi>, error out=w995:errorcluster)  [unwired: 3 in]
                n607 = call-by-ref "开始异步调用"(reference=w1000, error in=w995, "CODMn量程切换"=w993) -> (reference out=w999:refnum<vi>, error out=w994:errorcluster)  [unwired: 10 in]
                n608 = Close Reference(reference=w999, error in (no error)=w994) -> ()  [unwired: 1 out]
              }
              frame "Run top level" {
              }
              frame "Running" {
              }
            }
          }
        }
      }
      event "平行样测试": Value Change {
        n609 = event-data() -> ()  [unwired: 1 in, 6 out]
        n610 = flat-sequence {
          tunnel: [w1006] -> w1004
          tunnel: [w1008] -> w1003
          tunnel: [w1007] -> w1002
          tunnel: w1001 -> [w1005]
          tunnel: w1004 -> [w1015]
          tunnel: w1003 -> [w1014]
          tunnel: w1002 -> [w1013]
          frame #0 {
            n611 = Cancel Notification(0:w1005) -> ()  [unwired: 1 in, 3 out]
            n612 = call "平行样启动流程对话框.vi"() -> ("启动模块"=w1006:cluster{"氨氮1":bool, "总磷1":bool, " COD1":bool}, "直接启动"=w1007:bool, "常规启动"=w1008:bool)  [unwired: 8 in, 1 out]
            "常规启动 2" <- w1008
            "直接启动 2" <- w1007
            "启动模块 2" <- w1006
          }
          frame #1 {
            n613 = Bundle By Name(cluster=T5 {"是否启用仪器"=FALSE, "CODMn"={"启动测量模式"={"测量模式"=enum."水样测量"}, "确定按钮"=TRUE}, "启动模块"={"氨氮1"=FALSE, "总磷1"=FALSE, " COD1"=FALSE}, "常规启动"=FALSE, "直接启动"=FALSE} ("参数"), "是否启用仪器"=TRUE, "启动模块"=w1015, "常规启动"=w1014, "直接启动"=w1013) -> (w1010:T5)
            "输出簇 2" <- w1010
            n614 = vi-ref "古田户外一体站流程平行样自动启动.vi"() -> (w1011:refnum<vi>)
            n615 = property class="VI"(reference=w1011) -> ("Name"=w1012:string, "Exec.State"=w1009:T15)  [unwired: 1 in, 2 out]
            n616 = case shown="\"Idle\"" w1009 {
              tunnel: w1012 -> [_ w1024]
              tunnel: w1010 -> [_ w1018]
              frame "Bad", Default {
              }
              frame "Idle" {
                n617 = Open VI Reference(type specifier VI Refnum (for type only)=refnum<vi> refnum ("类型说明符VI引用句柄（仅用于类型）"), vi path=w1024, options=128 ("选项")) -> (vi reference=w1025:refnum<vi>, error out=w1023:errorcluster)  [unwired: 3 in]
                n618 = call-by-ref "开始异步调用"(reference=w1025, error in=w1023, "参数"=w1018) -> (reference out=w1020:refnum<vi>, error out=w1019:errorcluster)  [unwired: 9 in]
                n619 = Close Reference(reference=w1020, error in (no error)=w1019) -> ()  [unwired: 1 out]
              }
            }
          }
        }
      }
      event "停止测量": Value Change {
        # "停止采配水、氨氮、总磷总氮、COD、质控"
        n620 = event-data() -> ()  [unwired: 1 in, 6 out]
        n621 = call "质控启动参数选择对话框.vi"() -> ("确定启动"=w1026:bool, "启动模块"=w1027:T3)  [unwired: 9 in, 1 out]
        n622 = case shown="真" w1026 {
          tunnel: w1027 -> [_ w1037]
          frame False {
          }
          frame True {
            n623 = Unbundle By Name(w1037) -> ("氨氮"=w1035:bool, "总磷"=w1034:bool, "总氮"=w1033:bool, "COD"=w1036:bool)
            n624 = Or(x=w1034, y=w1033) -> (x .or. y?=w1032:bool)
            n625 = case shown="真" w1036 {
              frame False {
              }
              frame True {
                n626 = call "CODMn停止命令 (子VI).vi"() -> ()  [unwired: 12 in]
                n627 = Obtain Notifier(name (unnamed)="CODMn" ("名称（未命名）"), notification data type=FALSE) -> (notifier out=w1063:refnum<notifier>)  [unwired: 2 in, 2 out]
                n628 = Send Notification(notification=TRUE ("通知"), notifier=w1063) -> ()  [unwired: 1 in, 2 out]
                n629 = call "单个写入.vi"("value"=u16 2, "address"=u16 103, "Slave ID"=u8 3) -> ()  [unwired: 8 in, 1 out]
              }
            }
            n630 = case shown="真" w1035 {
              frame False {
              }
              frame True {
                n631 = Obtain Queue(name (unnamed)="NH3N" ("名称（未命名）"), element data type=cluster{"命令":string, "data":variant} {"命令"="", "data"=variant}) -> (queue out=w1059:refnum<queue>)  [unwired: 3 in, 2 out]
                n632 = Enqueue Element(queue=w1059, element=cluster{"命令":string, "data":variant} {"命令"="启动", "data"=variant(cluster{"站号":u16, "控制命令输出":u16[]} {"站号"=1, "控制命令输出"=[2816]})} ("元素")) -> ()  [unwired: 2 in, 3 out]
                n633 = Obtain Notifier(name (unnamed)="NH3N" ("名称（未命名）"), notification data type=FALSE) -> (notifier out=w1055:refnum<notifier>)  [unwired: 2 in, 2 out]
                n634 = Send Notification(notification=TRUE ("通知"), notifier=w1055) -> ()  [unwired: 1 in, 2 out]
                n635 = call "单个写入.vi"("value"=u16 2, "address"=u16 103, "Slave ID"=u8 1) -> ()  [unwired: 8 in, 1 out]
              }
            }
            n636 = case shown="真" w1032 {
              frame False {
              }
              frame True {
                n637 = Obtain Queue(name (unnamed)="TP" ("名称（未命名）"), element data type=cluster{"命令":string, "data":variant} {"命令"="", "data"=variant}) -> (queue out=w1048:refnum<queue>)  [unwired: 3 in, 2 out]
                n638 = Enqueue Element(queue=w1048, element=cluster{"命令":string, "data":variant} {"命令"="启动", "data"=variant(cluster{"站号":u16, "控制命令输出":u16[]} {"站号"=1, "控制命令输出"=[2816]})} ("元素")) -> ()  [unwired: 2 in, 3 out]
                n639 = Obtain Notifier(name (unnamed)="TNTP" ("名称（未命名）"), notification data type=FALSE) -> (notifier out=w1044:refnum<notifier>)  [unwired: 2 in, 2 out]
                n640 = Send Notification(notification=TRUE ("通知"), notifier=w1044) -> ()  [unwired: 1 in, 2 out]
                n641 = call "单个写入.vi"("value"=u16 2, "address"=u16 103, "Slave ID"=u8 2) -> ()  [unwired: 8 in, 1 out]
              }
            }
          }
        }
        n642 = Send Notification(notification=TRUE ("通知"), notifier=w1031) -> ()  [unwired: 1 in, 2 out]
        n643 = Enqueue Element At Opposite End(queue=w1028, element=T14 {"命令"="单个写入", {"starting address"=300, "holding register value"=2}} ("元素")) -> ()  [unwired: 2 in, 3 out]
      }
      event "查看": Value Change {
        n644 = event-data() -> ()  [unwired: 1 in, 6 out]
        n645 = property on="窗格" class="Pane"("Origin"=T7 {"Horizontal"=0, "Vertical"=600} ("原点")) -> ()  [unwired: 2 in, 2 out]
      }
      event "返回": Value Change {
        n646 = event-data() -> ()  [unwired: 1 in, 6 out]
        n647 = property on="窗格" class="Pane"("Origin"=T7 {"Horizontal"=0, "Vertical"=0} ("原点")) -> ()  [unwired: 2 in, 2 out]
      }
    }
  }
  n648 = Build Array("时间" ("table"), "参数" ("table"), "加标前水样测试时间" ("table"), "加标前水样浓度值" ("元素"), "加标后水样浓度值" ("元素"), "加标母液浓度值" ("元素"), "加标体积" ("元素"), "加标水杯定容体积" ("元素"), "加标回收率" ("元素")) -> (→"columns":string[])
  n649 = local write "背隙补偿步数 2"(w81) -> ()
  n650 = call-poly <vilib>:"Read Key.vi"("section"=w88, "error in (no error)"=w83, "key"="背隙值3", "refnum"=w84) -> ("error out"=w77:errorcluster, "value"=w79:i32, "refnum out"=w78:T13)  [unwired: 4 in, 1 out]
  n651 = local write "背隙补偿步数 3"(w79) -> ()
  n652 = call-poly <vilib>:"Read Key.vi"("section"=w70, "error in (no error)"=w77, "key"="标准体积1", "refnum"=w78) -> ("error out"=w73:errorcluster, "value"=w75:dbl, "refnum out"=w74:T13)  [unwired: 4 in, 1 out]
  n653 = local write "标准体积 1"(w75) -> ()
  n654 = call-poly <vilib>:"Read Key.vi"("section"=w70, "error in (no error)"=w73, "key"="标准体积2", "refnum"=w74) -> ("error out"=w71:errorcluster, "value"=w64:dbl, "refnum out"=w72:T13)  [unwired: 4 in, 1 out]
  n655 = local write "标准体积 2"(w64) -> ()
  n656 = call-poly <vilib>:"Read Key.vi"("section"=w70, "error in (no error)"=w71, "key"="标准体积3", "refnum"=w72) -> ("error out"=w68:errorcluster, "value"=w63:dbl, "refnum out"=w69:T13)  [unwired: 4 in, 1 out]
  n657 = local write "标准体积 3"(w63) -> ()
  n658 = call-poly <vilib>:"Read Key.vi"("section"=w70, "error in (no error)"=w68, "key"="标准体积4", "refnum"=w69) -> ("error out"=w66:errorcluster, "value"=w48:dbl, "refnum out"=w67:T13)  [unwired: 4 in, 1 out]
  n659 = local write "标准体积 4"(w48) -> ()
  n660 = call-poly <vilib>:"Read Key.vi"("section"=w70, "error in (no error)"=w66, "key"="标准体积5", "refnum"=w67) -> ("error out"=w57:errorcluster, "value"=w47:dbl, "refnum out"=w58:T13)  [unwired: 4 in, 1 out]
  n661 = local write "标准体积 5"(w47) -> ()
  n662 = call-poly <vilib>:"Read Key.vi"("section"=w70, "error in (no error)"=w57, "key"="实际体积1", "refnum"=w58) -> ("error out"=w55:errorcluster, "value"=w46:dbl, "refnum out"=w56:T13)  [unwired: 4 in, 1 out]
  n663 = local write "实际体积 1"(w46) -> ()
  n664 = call-poly <vilib>:"Read Key.vi"("section"=w70, "error in (no error)"=w55, "key"="实际体积2", "refnum"=w56) -> ("error out"=w53:errorcluster, "value"=w45:dbl, "refnum out"=w54:T13)  [unwired: 4 in, 1 out]
  n665 = local write "实际体积 2"(w45) -> ()
  n666 = call-poly <vilib>:"Read Key.vi"("section"=w70, "error in (no error)"=w53, "key"="实际体积3", "refnum"=w54) -> ("error out"=w51:errorcluster, "value"=w42:dbl, "refnum out"=w52:T13)  [unwired: 4 in, 1 out]
  n667 = local write "实际体积 3"(w42) -> ()
  n668 = call-poly <vilib>:"Read Key.vi"("section"=w70, "error in (no error)"=w51, "key"="实际体积4", "refnum"=w52) -> ("error out"=w49:errorcluster, "value"=w41:dbl, "refnum out"=w50:T13)  [unwired: 4 in, 1 out]
  n669 = call-dynamic "Close Session.vi"("error in (no error)"=w137, "MB_Serial session"=w97) -> ()  [unwired: 9 in, 1 out]
  n670 = local write "实际体积 4"(w41) -> ()
  n671 = call-poly <vilib>:"Read Key.vi"("section"=w70, "error in (no error)"=w49, "key"="实际体积5", "refnum"=w50) -> ("error out"=w36:errorcluster, "value"=w40:dbl, "refnum out"=w37:T13)  [unwired: 4 in, 1 out]
  n672 = local write "实际体积 5"(w40) -> ()
  n673 = call-poly <vilib>:"Read Key.vi"("section"="质控手动体积选择", "error in (no error)"=w36, "key"="手动体积选择" ("section"), "refnum"=w37) -> ("error out"=w30:errorcluster, "value"=w33:i32, "refnum out"=w31:T13)  [unwired: 4 in, 1 out]
  n674 = local write "注出体积选择"(w33) -> ()
  n675 = call-poly <vilib>:"Read Key.vi"("section"=w32, "error in (no error)"=w30, "key"="模块1" ("section"), "refnum"=w31) -> ("error out"=w28:errorcluster, "value"=w20:bool, "refnum out"=w29:T13)  [unwired: 4 in, 1 out]
  n676 = call-poly <vilib>:"Read Key.vi"("section"=w32, "error in (no error)"=w28, "key"="模块2" ("section"), "refnum"=w29) -> ("error out"=w26:errorcluster, "value"=w21:bool, "refnum out"=w27:T13)  [unwired: 4 in, 1 out]
  n677 = local write "模块选择"(w20) -> ()
  n678 = local write "模块选择 2"(w21) -> ()
  n679 = call-poly <vilib>:"Read Key.vi"("section"=w32, "error in (no error)"=w26, "key"="模块3" ("section"), "refnum"=w27) -> ("error out"=w18:errorcluster, "value"=w22:bool, "refnum out"=w19:T13)  [unwired: 4 in, 1 out]
  n680 = local write "模块选择 3"(w22) -> ()
  n681 = call-poly <vilib>:"Read Key.vi"("section"=w17, "error in (no error)"=w18, "key"="氨氮" ("section"), "refnum"=w19) -> ("error out"=w15:errorcluster, "value"=w4:u32, "refnum out"=w16:T13)  [unwired: 4 in, 1 out]
  n682 = local write "氨氮量程选择"(w4) -> ()
  n683 = call-poly <vilib>:"Read Key.vi"("section"=w17, "error in (no error)"=w15, "key"="总氮" ("section"), "refnum"=w16) -> ("error out"=w13:errorcluster, "value"=w3:u32, "refnum out"=w14:T13)  [unwired: 4 in, 1 out]
  n684 = local write "总氮量程选择"(w3) -> ()
  n685 = call-poly <vilib>:"Read Key.vi"("section"=w17, "error in (no error)"=w13, "key"="总磷" ("section"), "refnum"=w14) -> ("error out"=w11:errorcluster, "value"=w2:u32, "refnum out"=w12:T13)  [unwired: 4 in, 1 out]
  n686 = local write "总磷量程选择"(w2) -> ()
  n687 = call-poly <vilib>:"Read Key.vi"("section"=w17, "error in (no error)"=w11, "key"="CODMn" ("section"), "refnum"=w12) -> ("error out"=w9:errorcluster, "value"=w1:u32, "refnum out"=w10:T13)  [unwired: 4 in, 1 out]
  n688 = local write "CODMn量程选择"(w1) -> ()
  n689 = call <vilib>:"Close Config Data.vi"("error in (no error)"=w9, "refnum"=w10) -> ()  [unwired: 8 in, 2 out]
  "VISA Resource" <- w96
  "Serial Config" <- w95
